vi "Doktorarbeit_Cornelius.vi"(0 "Heizer":refnum<visa-resource-name>="COM1", 1 "Setpoint\n START":bool, 2 "Write to File":bool, 3 "SP 1 shall be (°C)":dbl=20.0 min=0.0 max=999.0, 4 "Intervall (s)":u32 max=600, 5 "Write/\nRead":bool=TRUE, 6 "Delay (ms)":u32=500 min=100 max=600000, 7 "Auto Tune":bool, 9 "Standby":bool, 11 "Reset\nSTOPP":bool, 12 "Read Temperature":bool=TRUE, 13 "Get Values":bool, 15 "File Path":path) -> (8 "Temperature (°C)":dbl format="%#.3f", 14 "SP 1 is (°C)":dbl)   [LabVIEW 2010]
doc: "1. Verwendung\n\nDas Programm dient der Steuerung und Abfrage des Thermocontrollers I3252 und dem Auslesen von zwei VC 840 Messgeräten und einem Druckmessgerät Pfeiffer Single Gauge. \nDie Messgeräte werden Standardmäßig ausgelesen und erst nach Betätigung des Schalters \"Write to File\" in einer Textdatei abgespeichert. Das Eingabefeld \"Intervall\" legt den Abstand der Messpunkte fest.\nDer Setpoint für den Thermocontroller wird erst nach Betätigung des Tasters \"Setpoint START\" übernommen und angesteuert. Er wird ind den EEPROM des Gerätes geschrieben. Die Regelung kann mit Hilfe des Schalters \"Standby\" unterbrochen werden. Durch den Taster \"Reset STOPP\" kann der Setpoint aus dem EEPROM gelöscht werden.\nDie Eingabeflächen \"Constant\" und \"Thickness\" dienen der Berechnung des spezifischen Widerstands.\nDie Eingabeflächen \"User\" und \"Sample\" werden in den Header der Textdatei übernommen.\nDer Indikator \"File Path\" zeigt den aktuellen Speicherort der Textdatei an. Dieser wird nach ausschalten des Schalters \"Write to File\" gelöscht. Bei erneuten Schreiben muss ein neuer Speicherort gewählt werden. Bei Wahl desselben Speicherorts werden sämtliche bereits gespeicherte Daten gelöscht.\n\n\n2. Erläuterungen zum Blockdiagramm\n2.1 äußere Sequenz\nDie äußerte Sequenz besteht aus fünf Frames. Der erste dient der Initialisierung der Ports. Der zweite dient als Verzögerung um dem Programm genug Zeit zu geben die Ports zu öffnen. Jedoch senden die beiden VC 840 bereits Informationen an den Computer die in einem Puffer zwischengespeichert werden. Im dritten Frame wird dieser Puffer geleert. Somit kommt es zu keinem Framing Error. Desweiteren wird in diesem Frame die Startzeit der Messungen genommen. Im vierten Frame wird die eigentliche Messung und Verarbeitung der Daten durchgeführt. Die while-Schleife wird nur durch Auftreten eines Fehlers oder durch Betätigung des Stopbuttons auf dem Front Panel in der oberen linken Ecke unterbrochen. Im fünften und letzten Frame werden die Ports wieder geschlossen und beim Auftreten eines Fehlers wird das Programm automatisch gestoppt. Falls kein Fehler auftritt wird die Sequenz von vorne abgearbeitet.\n\n2.2 while-Schleife und innere Sequenz\n2.2.1 \"Event Structure\"\n2.2.1.1 Allgemein\nDer erste Frame beinhaltet ein \"Event Structure\". Dieser reagiert auf insgesamt elf verschiedene Ereignisse. Falls keines dieser Ereignisse auftreten sollte, warte die Struktur eine Millisekunde bevor die \"Event Structure\" verlassen wird. Die übrigen Ereignisse treten ein, wenn der entsprechende Kontroller eine Werteänderung erfährt.\n\n2.2.1.2 Event: Setpoint\nDieser Case besteht von außen nach innen aus einer Stacked Sequence, einer for-Loop und einer Flat Sequence die wiederum zwei \"Case Structures\" enthält. Als erstes wird bei dem Schalter \"Setpoint START\" der Blinkmodus aktiviert und bei dem Schalter \"Read Temperature\" deaktiviert. Danach folgt das eigentliche setzen des Temperatursollwerts. In der ersten Iteration wird dem Controller I3252 ein Schreibbefehl gesendet. Theoretisch kann der Setpoint in den RAM oder in den EEPROM geschrieben werden. Diese Auswahl erfolgt mit Hilfe des Schalters \"RAM\". Da das Schreiben in den RAM -Speicher aber aus diversen Gründen nicht erwünscht ist, wurde es nicht implementiert. Eine nachträgliche Implementierung ist aber leicht möglich, in dem die untere String-Konstante \"*P012\" durch \"*W012\" ersetzt wird. An diesem Befehl wird eine fünfstellige Hexadezimalzahl angehängt, die den Sollwert wiedergibt. Der Sollwert wird vorher mit zehn multipliziert, da das Komma standardmäßig nach der ersten Ziffer festgesetzt wurde (Bsp.: 800 wird gesendet um 80 einzustellen). Dieser Befehlsstrang wird an das Gerät mittels des SubVIs \"Comm_Interface\", auf welches später noch näher eingegangen wird, weitergegeben. Der durch das Gerät zurückgegebene String wird nicht verarbeitet.\nDie zweite Iteration dient dem Auslesen des eingestellten Sollwertes. Wahlweise kann der RAM- oder der EEPROM-Speicher ausgelesen werden. Die eigentliche Verarbeitung des Ausgabestrings erfolgt durch das SubVI \"Edit Setpoint\".\nDie Implementierung zur Einstellung des zweiten Setpoints erfolgt durch kopieren der ersten beiden Fälle und ersetzen der \"1\" im Befehf durch eine \"2\" (Bsp.: \"*P012\" zu \"*P022\"). Es darf aber nicht vergessen werden, dass dann ebenfalls die Anzahl der Iterationen angepasst werden muss.\nAls letztes wird der Blinkmodus des Schalters \"Setpoint START\" wieder deaktiviert.\n\n2.2.1.3 Event: Standby\nDieses Ereignis aktiviert bzw. deaktiviert als erstes den Blinckmodus des entsprechenden Schalters und sendet danach den Befehl zum aktivieren (\"*D03\") oder zum deaktivieren (\"*E03\") des Standbymodus an den Thermocontroller.\n\n2.2.1.4 Event: Set Command \nDer in das Feld \"Command shall be\" eingegebene Befehl wird an den Thermocontroller übermittlet. Die korrekte Form des Befehls ist im \"Communication Manuel\" nachzuschlagen. Das \"*\"-Zeichen wurde allerdings schon implementiert und muss somit nicht mit eingegeben werden.\n\n2.2.1.5 Event: Reset\nIn der ersten Iteration wird der Reset-Befehl an den Thermocontroller gesendet. In Folge wird der gesamte EEPROM-Speicher gelöscht. Deshalb wird in der zweiten Iteration der Setpoint aktualisiert. Dieser Befehl hat keinen Einfluss auf den RAM-Speicher. Die anschließende Wartezeit ist auf vier Sekunden festgesetzt und wurde empirisch ermittelt. Diese Zeit benötigt das Gerät um den Reset durchzuführen und für die Kommunikation wieder zur Verfügung zu stehen.\n\n2.2.1.6 Event: Auto Tune\nEs ist festgeschrieben, dass der Setpoint für die \"Auto Tune\"-Funktion wenigstens 20°C über der aktuellen Temperatur liegt. Deshalb wird zunächst der aktuelle Temperaturwert ausgelesen. Im zweiten Schritt werden zu diesem Wert zwanzig addiert und der Setpoint wird in den RAM-Speicher geschrieben. Das Schreiben in diesen Speicher ist nötig, da die \"Auto Tune\"-Funktion\" erst nach einem Reset startet. Im dritten Schritt wird der eigentliche Befehl für den \"Auto Tune\" gesendet (siehe dazu \"Communication Manuel\" S.27). Als vierte und letzte Iteration der for-Schleife folgt der bereits erwähnte Reset-Befehl. Der Temperatursollwert, der im RAM-Speicher eingetragen ist, muss zum Schluss wieder auf 0°C gesetzt werden. Die Zeit für die Ausführung des \"Auto Tune\"-Befehls wurde empirisch ermittelt und 45 s festgesetzt.\n\n2.2.1.7 Event: Write LOW/HI\nDieses Ereignis setzt die am Analogausgang anliegende Spannung fest. Normalerweise beträgt dieser Spannungswert 0-10 V. Das angeschlossene Netzteil verträgt aber maximal nur 2,3 V. Aus diesem Grund wird der \"%HIGH\" auf 23 gesetzt. Somit beträgt die maximal anliegende Spannung nur noch 23% von der maximal möglichen, d.h 2,3V. Ein niedrigerer Wert ist jederzeit möglich, genauso wie ein höherer für den Parameter \"%LOW\". Diese werden zunächst nacheinander in den RAM-Speicher geschrieben und anschließend wieder ausgelesen.\n\n2.2.1.8 Event: Set PID\nDie Werte für den PID-Regler können sowohl mit Hilfe der \"Auto Tune\"-Funktion, als auch manuell eingestellt werden. Es wird wiederum zwischen dem Schreiben in den RAM- und dem EEPROM-Speicher unterschieden. Zunächst werden die Werte für \"P\", \"I\" und \"D\", in dieser Reihenfolge, gesetzt und danach die aktuellen Werte ausgelesen.\n\n2.2.1.9 Event: Get Values\nDieses Ereignis hat zur Folge, dass die Werte für \"P\", \"I\", \"D\", \"%LOW\", \"%HIGH\" und des Setpoints wahlweise aus dem RAM- oder EEPROM-Speicher gelesen werden. Die aktuellen Werte werden nicht nur in die entsprechenden Anzeigefelder übernommen, sondern auch in die entsprechenden Eingabefelder, mit Ausnahme des Temperatursollwerts. \n\n2.2.1.10 Event: RAM\nPrinzipiell kann zwischen dem Schreiben in den RAM- oder EEPROM-Speicher des Thermocontrollers gewählt werden. Die entsprechende Schalterposition auf dem Frontpanel zeigt den aktuell verwendeten Speicher an. Die Anzeigewerte werden bei jedem Umschalten aktualisiert und sind im entsprechenden Speicher eingetragen. Die Implementierung ist identisch mit der des Ereignisses \"Get Values\". Es gilt zu beachten, dass die Werte für \"%LOW\" und \"%HIGH\" nur in den RAM-Speicher geschrieben werden können und somit auch nur aus diesem ausgelesen werden können.\n\n2.2.1.11 Event: Set Gauge to Zero\nMit Hilfe der SubVIs \"Get Pressure\" und \"Offset Display\" werden die Werte für den alten und den neuen Offset und der durch den zweiten Drucksensor ermittelt Druck ermittelt. \n\n2.2.1.12 Event: Write to File\nSollte der Schalter \"Write to File\" aktiviert werden, d.h. Schalterposition oben, so wird zunächst durch das SubVI \"Header\" ein Header für die unter \"File Path\" definierte Datei angelegt. Alle Werte, die bereits in der entsprechenden Datei stehen, werden dabei gelöscht.\n\n2.2.2 \"Timed Structures\"\nIm dritten Frame der inneren Sequenz werden die Werte für Zeitpunkt, Temperatur, Spannung, Strom und Druck ermittelt. Damit die Werte zum gleichen Zeitpunkt aufgenommen werden, werden \"Timed Sequences\" eingesetzt. Mit dem entsprechenden Schalter auf dem Front Panel unter dem Tab \"Settings\" kann gewählt werden, ob das entsprechende Gerät ausgelesen werden soll oder nicht. Die einzelnen Sequenzen werden parallel abgearbeitet, womit die Prozesszeit von diesem Frame durch der zeitintensivsten Sequenz abhängt. Dies ist in aller Regel das Auslesen der Temperatur, da ein \"Delay\" von 500 ms oder größer benötigt wird, um den Controller ordentlich ansprechen zu können.\nDie Systemzeit wird durch das SubVI \"System Time in Seconds\" in Sekunden umgerechnet und der in dem Parameter \"Starttime\" gespeicherte Wert wird abgezogen. Somit werden die Sekunden seit dem Start des Programms gezählt.\n\n2.2.3 restlichen Frames\nIm zweiten Frame wird das Intervall zwischen den einzelnen Messwerten festgelegt. Dabei wird der Wert des Parameters \"Delay\" abgezogen. Dieser Wert beträgt im Normalfall 500 ms und ist somit nicht vernachlääsigbar.\nDer Vierte Frame beinhaltet die Umrechnung des Temperatur-Strings in einen Temperaturwert durch das SubVI \"Edit Tmperature\", die Berechnung des spezifischen Widerstands durch das SubVI \"Resistivity Calculation\" und die Überprüfung des Druckwerts. Auch werden die neu gewonnen Werte in das entsprechende Shift-Register übernommen. Falls der Druckwert einen in dem Parameter \"Pressure Limit (mbar)\" festgelegten Grenzwert überschreiten sollte, wird der Thermocontroller automatisch in den Standby-Modus versetzt. Des Weiteren wird der Schalter \"Standby\" solange gesperrt, wie der Druck oberhalb des Grenzwertes liegt. Wenn der Druck wieder unter den Grenzwert gesunken ist, wird der Standby-Befehl nicht automatisch aufgehoben, sondern muss vom Benutzer durch Betätigung des entsprechenden Schalters gegeben werden.\nIm fünften Frame werden die Diagramme erstellt. Dabei wird jedes Mal von neuem das gesamte Shift-Register als Graph dargestellt. Weiterhin werden die Messwerte in ein 1D-Array geschrieben.\nDer sechste und letzte Frame beinhaltet den eigentlich Schreibvorgang der Messwerte in eine Textdatei und die Überprüfung ob ein Fehler vorliegt.\n\n2.3 SubVIs\n2.3.1 Allgemein\nDie SubVIs für die Messgeräte VC840 und das Druckmessgerät wurden aus anderen Quellen übernommen. \n\n2.3.2 \"Header\"\nIn den Header wird zunächst das aktuelle Datum und die aktuelle Zeit übernommen. Die ausgewählte Datei wird dabei überschrieben. Danach wird der Name des Benutzers und der Probe übernommen. Zum Schluss werden die Einheiten in einer Reihe, durch einen Tabulator getrennt, in den Header geschrieben.\n\n2.3.3 \"I3252 Comm Interface\"\nDieses VI stellt die Kommunikation mit dem Thermocontroller her und gibt den Ausgabe-String zurück.\n\n2.3.4 \"I3252 Edit Setpoint\"\nIm Ausgabe-String vom Thermocontroller ist an der vierten Stelle die Stelle des Dezimalpunktes verschlüsselt. Dieses Hexadezimalzahl wird herausgefiltert und an ein \"ENUM Controller\" übergeben. Dieser weist der Hexadezimalzahl eine Nummer zu, mit welcher ein Wert aus einem Array entnommen wird. Dieser Wert dient als Quotient. Der tatsächliche Wert kann somit errechnet werden.\n\n2.3.5 \"I3252 Edit Temperature\"\nDer Temperatur-String, der vom Thermocontroller zurückgegeben wird, wird in eine Dezimalzahl umgewandelt. Manchmal kommt es aus zu Dropouts, die durch dieses Programm herausgefiltert werden. Der letzte Wert wird dabei in einer \"Feedback Node\" gehalten unter der Annahme, dass sich der Temperaturwert nicht sprunghaft ändert.\n\n2.3.6 \"Resistivity Calculation\"\nDer spezifische Widerstand wird nach folgender Formel ausgerechnet. Dabei entspricht t der Dicke der Probe und C ist eine Konstante.\nrho=C*pi*t*U/(ln( 2)*I)\n\n2.3.7 \"System Time in Seconds\"\nZunächst wird die aktuelle Systemzeit ausgelesen. Danach wird diese in Stunden, Minuten und Sekunden aufgeteilt, alles in Sekunden umgerechnet und letztendlich addiert."
uses:
  <vilib>/Platform/TimedLoop/XDataNode/XDataNode.xnode
  <vilib>/Platform/TimedLoop/XDataNode/timing_clust.ctl
  <vilib>/Platform/TimedLoop/XDataNode/nitl_modes.ctl
  <vilib>/Platform/TimedLoop/XDataNode/wakeup.ctl
  <vilib>/Instr/_visa.llb/VISA Configure Serial Port (Instr).vi
  <vilib>/Platform/TimedLoop/scheduler/LVUserAPI/_suppVIs/Create_1kHz_TSource.vi
  <vilib>/Utility/file.llb/Write To Spreadsheet File (DBL).vi
  <vilib>/Platform/TimedLoop/XDataNode/XDNodeRunTimeDep.lvlib
panel:
  out "appended array":dbl[](array[numeric])
  in  "Tab Control":T1(tab)
  out "Pressure":cluster{dbl[], dbl[]}(graph)
  out "Pressure (mbar)":dbl format="%.2e"
  in  "Thickness (nm)":dbl min=0.0
  in  "Constant":dbl=4.532 min=0.0 max=5.0
  in  "Sample":string
  in  "User":string
  out "Temperature":cluster{dbl[], dbl[]}(graph)
  out "Resistivity":cluster{dbl[], dbl[]}(graph)
  out "Resistivity (Ohm*cm)":dbl format="%.3e"
  out "time (s)":dbl
  in  "Pressure Limit (mbar)":dbl=0.0001 min=0.0 max=1100.0
  out "Pressure 1 (mbar)":dbl
  out "Current Offset (mbar)":dbl
  out "Old Offset (mbar)":dbl
  out "Pressure 2 (mbar)":dbl
  out "Status":T2(ring)
  in  "Sensor Nr.:":enum16{"sensor 1", "aensor 2", "test"}(ring)
  in  "Port":T3(ring)=enum."COM 5"
  in  "Set Gauge to Zero":bool
  out "Error Out":bool
  in  "VC 840 2":refnum<visa-resource-name>="COM4"
  out "Reading 2":dbl format="%_4f"
  out "Mode 2":enum16{"?", "Diode", "Beep", "DC", "AC"}(ring)
  out "Unit 2":string
  in  "VC 840 1":refnum<visa-resource-name>="COM3"
  out "Reading 1":dbl format="%_4f"
  out "Mode 1":enum16{"?", "Diode", "Beep", "DC", "AC"}(ring)
  out "Unit 1":string
  out "Status 1":T4
  out "Status 2":T4
  in  "Set Command":bool
  in  "Set PID":bool
  in  "Write LOW/HI":bool
  out "% HIGH is":u32
  out "% LOW is":u32
  in  "% High shall be":u32=23 max=24
  in  "% LOW shall be":u32 max=25
  in  "Flow Control":u16(ring) items=["None"=0, "XON/XOFF"=1, "RTS/CTS"=2, "DTR/DSR"=4]
  in  "Stop Bits":u16(ring)=10 items=["1.0"=10, "1.5"=15, "2.0"=20]
  in  "Parity":u16(ring)=1 items=["None", "Odd", "Even", "Mark", "Space"]
  in  "Data Bits":u16=7 min=5 max=8 step=1
  in  "Baud Rate":u32=9600
  out "Command is":string
  in  "Command shall be":string
  in  "RAM":bool=TRUE caption="EEPROM"
  out "D (Rate) is":u32
  out "I ( Reset1) is":u32
  out "P (PB1) is":u32
  in  "D (Rate) shall be":u32 max=3999
  in  "I ( Reset1) shall be":u32 max=3999
  in  "P (PB1) shall be":u32 max=9999
  in  "Read VC 840 1":bool=TRUE
  in  "Read VC 840 2":bool=TRUE
  in  "Read Pressure":bool=TRUE
  out "Starttime":dbl
  out "Current":cluster{dbl[], dbl[]}(graph)
  out "Voltage":cluster{dbl[], dbl[]}(graph)
  out "Voltage (V)":dbl format="%.4e"
  out "Current (A)":dbl format="%.4e"
  # "I3252 Control"
  # "VC 840 Control"
  # "Pfeiffer Control"
  # "Authors:  Daniel Schuster (sir-dan@web.de)\n                 Steffen Cornelius (s.cornelius@hzdr.de)\n\n                 premade SubVIs for readout of Pfeiffer gauge and VC840 Multimeters were used\n                 SubVI \"I3252_Comm_Interface\" is based on a modified Labview example\n\nRelease:  v1.0    \n\nVersion History:\n\nv1.1  28.06.2011\n             - Format des Files geändert von %.3f auf %g\n             - maximale Eingabewerte für PID begrenzt\nv1.2  12.07.2011\n             - Anzeige p,rho, U, V auf Scientific geändert\n             - y-Achse p,rho auf Log geändert\n             - numerische Zeitanzeige hinzugefügt\n             - 4PP Constant: pi/ln(2)=4,532 set as the default value\nv1.3  25.07.2011\n             - Zeitvariable auf EXT geändert, um Sprünge in Diagrammen loszuwerden"
  # "Version 1.3    - last change 25.07.2011"
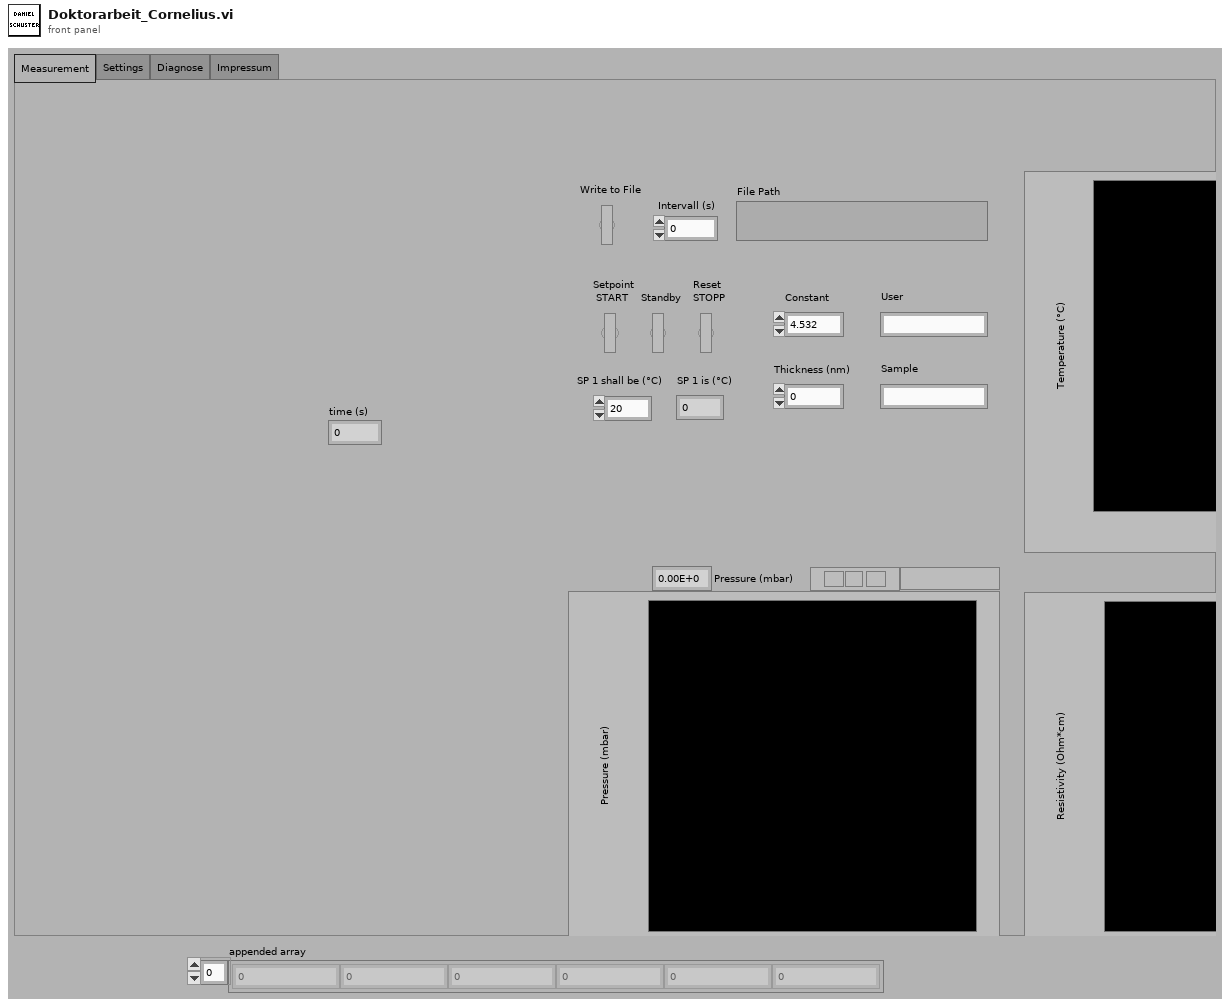
[diagram p1: front panel]
types:
  T1 = enum32{"Measurement", "Settings", "Diagnose", "Impressum"}
  T2 = enum16{"data OK", "underrange", "overrange", "sensor error", "sensor off", "no sensor", "ID error"}
  T3 = enum16{"COM 1", "COM 2", "COM 3", "COM 4", "COM 5", "COM 6", "COM 7", "COM 8", "COM 9", "COM 10", "COM 11", "COM 12"}
  T4 = cluster{"Low Bat":bool, "Auto":bool, "Delta":bool, "Hold":bool, "RS232":bool}
  T5 = typedef "XDNodeRunTimeDep.lvlib/timing_clust.ctl" = cluster{"Expected End [f-1]":u64, "Actual End [f-1]":u64, "Finished Late? [f-1]":bool, "Expected End [i-1]":u64, "Actual End [i-1]":u64, "Finished Late? [i-1]":bool, "Expected Start [i]":u64, "Actual Start [i]":u64, "Expected Start [f]":u64, "Actual Start [f]":u64, "Source Name":string, "Structure Name":string, "Period":i64, "Deadline":i64, "Offset":i64, "Start":i64, "Priority":i32, "Timeout":i32, "Mode":T6, "Wakeup Reason":T7, "Error":errorcluster, "Source Type":string, "Secondary Source Type":string, "Global End Time":u64, "Global Start Time":u64, "Frame Duration":u64, "Iteration Duration":u64, "Assigned CPU":i32, "I/O Scan Engine Mode":u32}
  T6 = typedef "XDNodeRunTimeDep.lvlib/nitl_modes.ctl" = enum32{"No Change", "Process missed periods, maintain original phase", "Discard missed periods, maintain original phase", "Process missed periods, ignore original phase", "Discard missed periods, ignore original phase"}
  T7 = typedef "XDNodeRunTimeDep.lvlib/wakeup.ctl" = enum32{"Normal", "Aborted", "Asynchronous wakeup", "Timing source error", "Timed loop error", "Timeout"}
  T8 = enum8{"Enabled", "Disabled", "Disabled and Grayed Out"}
  T9 = cluster{"VISA resource name out":refnum<visa-resource-name>, "error out":errorcluster, "Delay (ms)":u32, "Write/\nRead":bool}
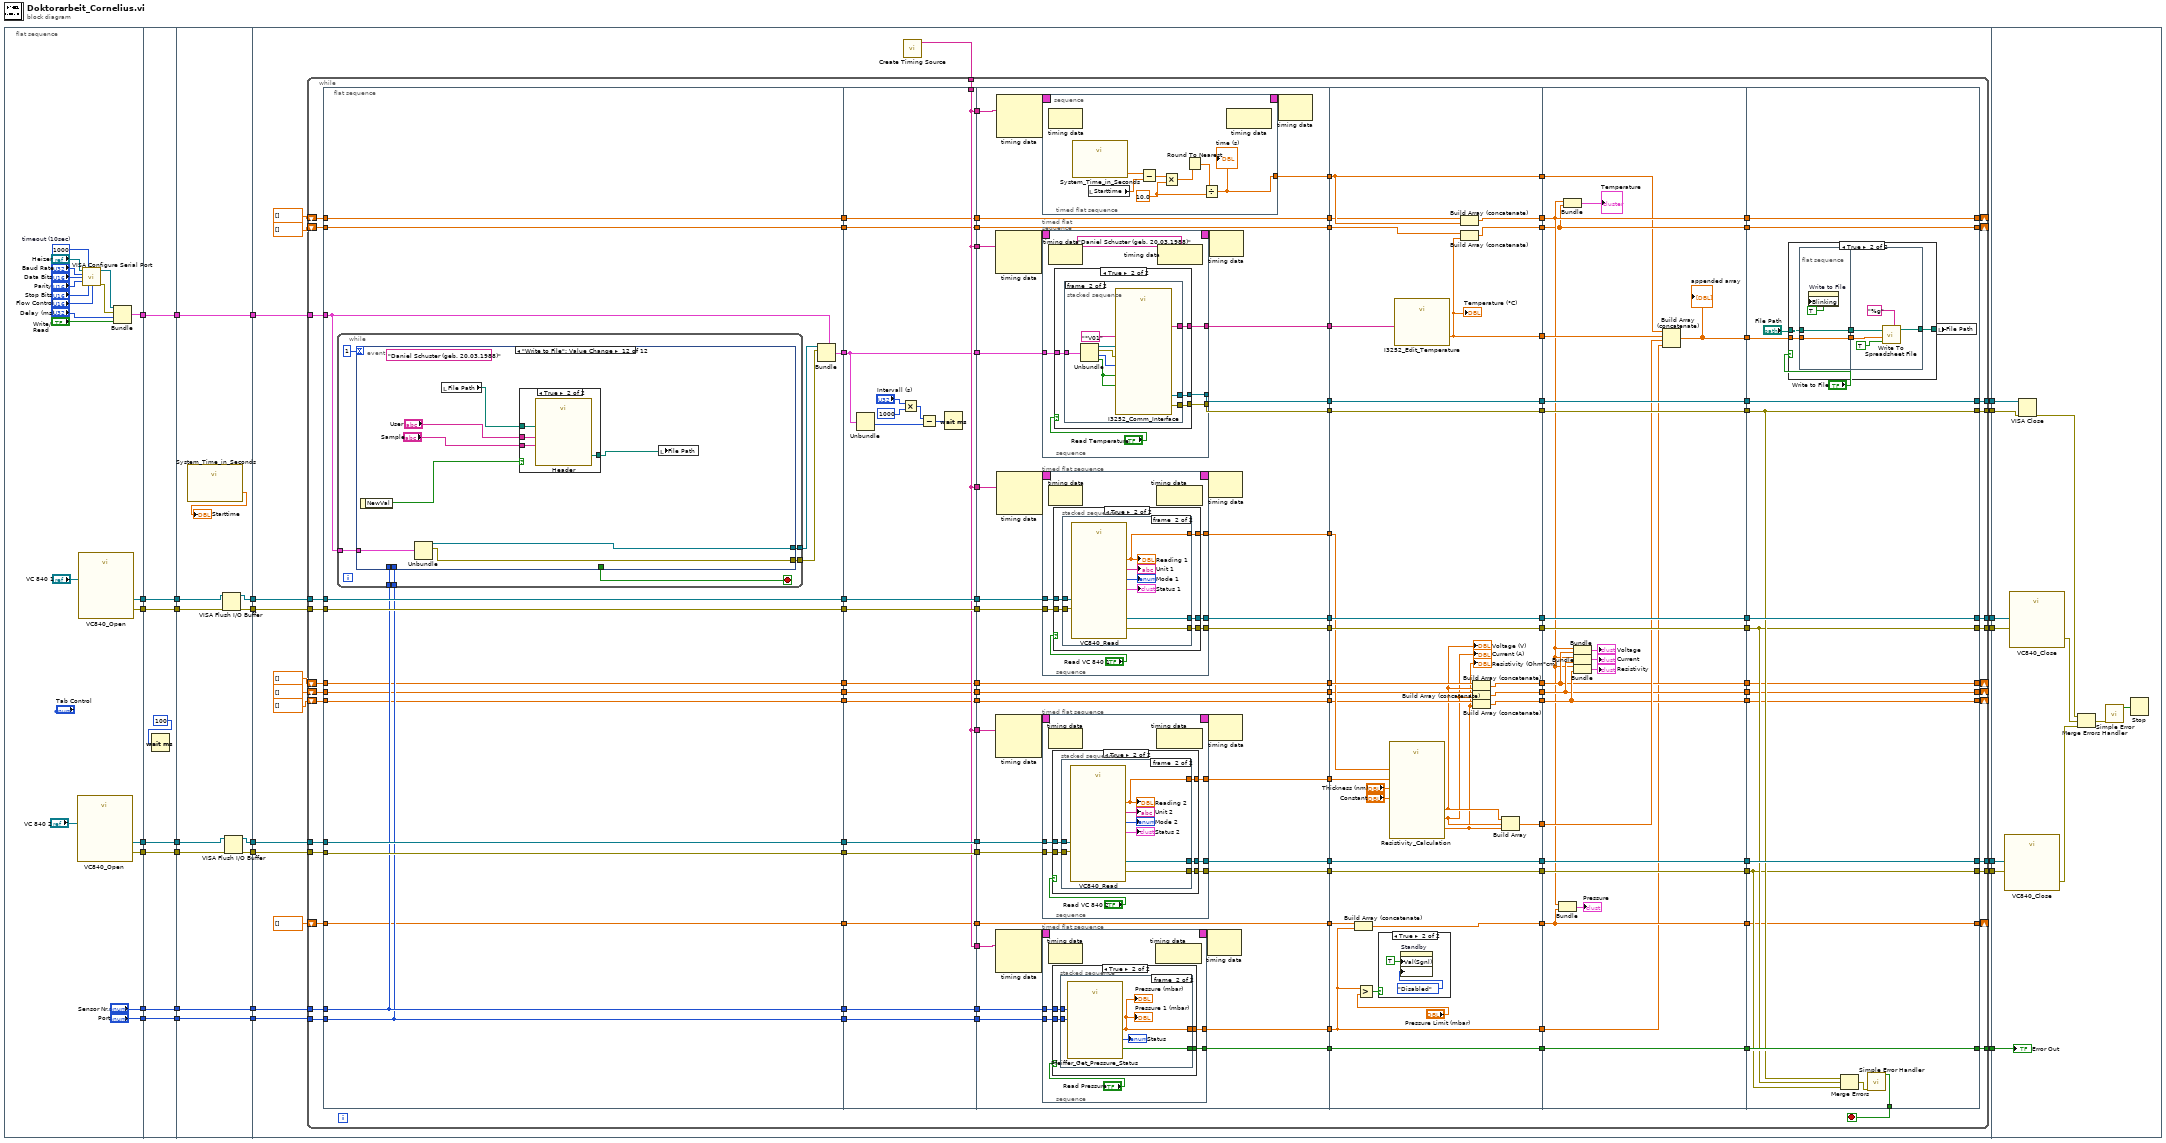
[diagram p0: block diagram]
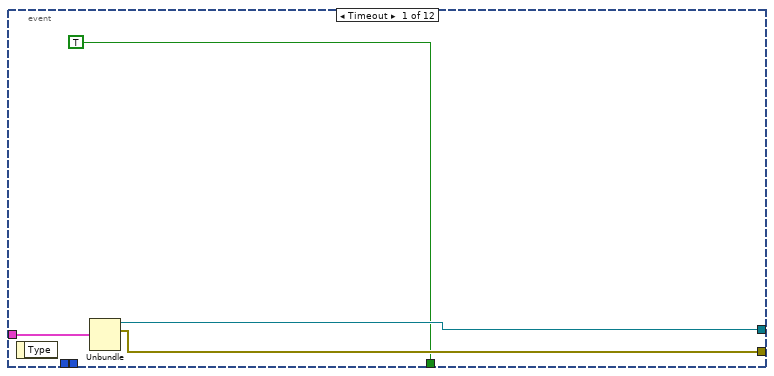
[diagram p2: hidden frame]
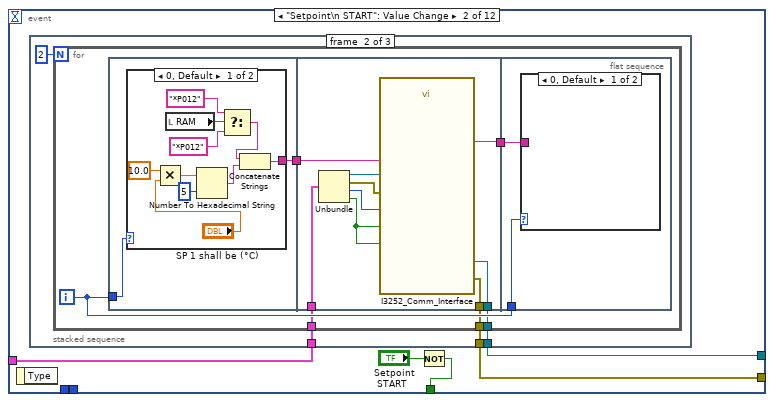
[diagram p3: hidden frame]
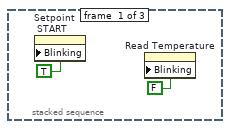
[diagram p4: hidden frame]
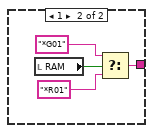
[diagram p5: hidden frame]
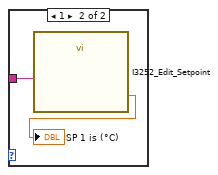
[diagram p6: hidden frame]
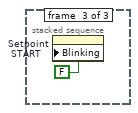
[diagram p7: hidden frame]
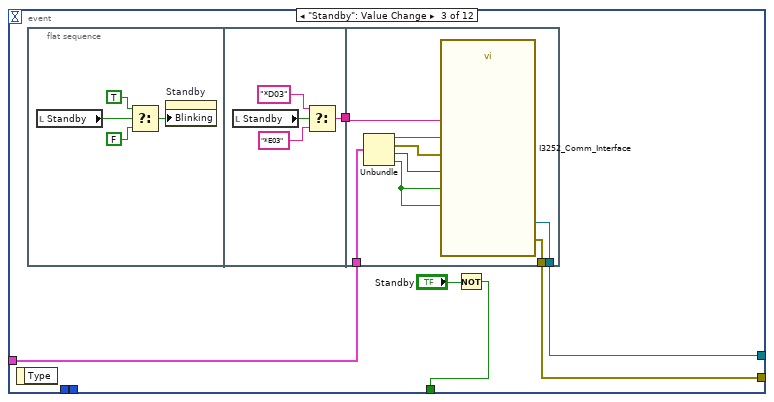
[diagram p8: hidden frame]
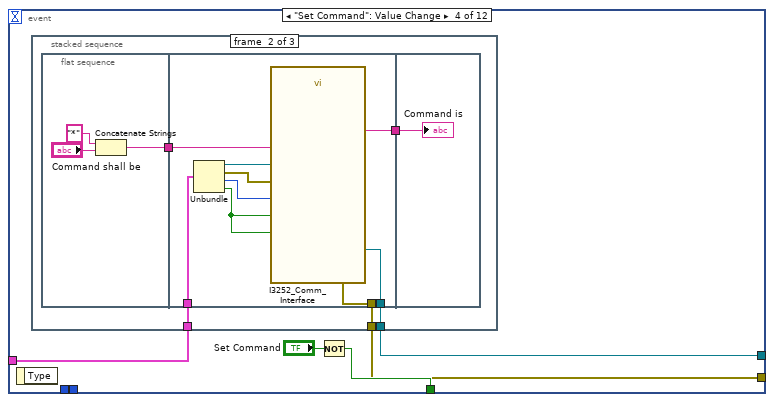
[diagram p9: hidden frame]
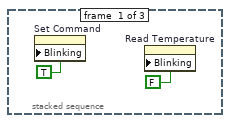
[diagram p10: hidden frame]
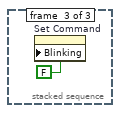
[diagram p11: hidden frame]
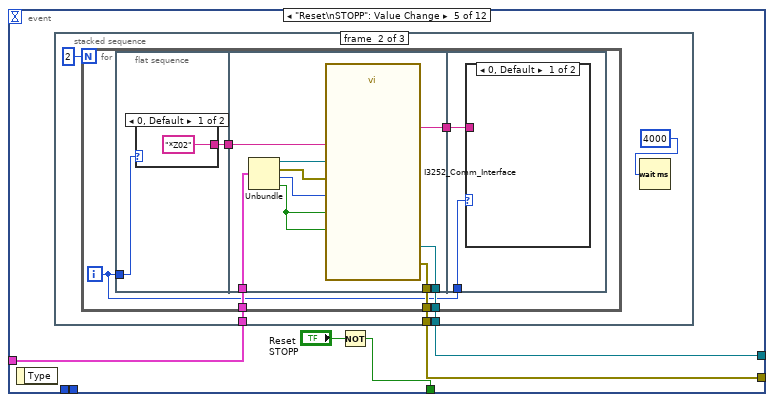
[diagram p12: hidden frame]
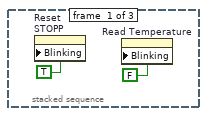
[diagram p13: hidden frame]
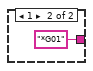
[diagram p14: hidden frame]
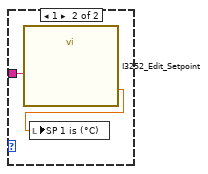
[diagram p15: hidden frame]
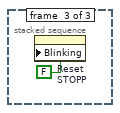
[diagram p16: hidden frame]
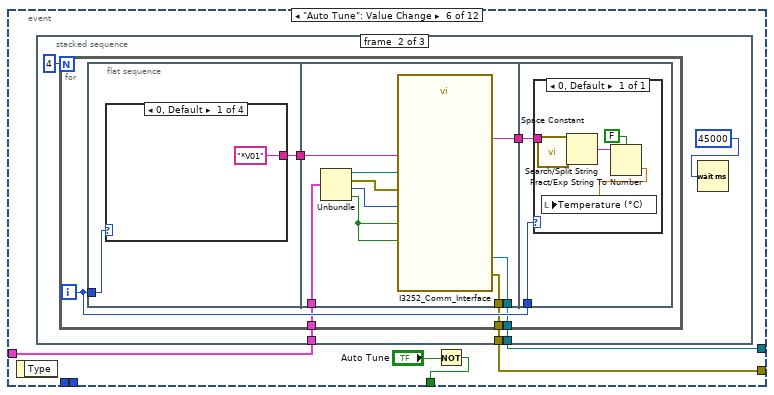
[diagram p17: hidden frame]
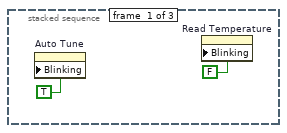
[diagram p18: hidden frame]
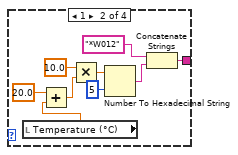
[diagram p19: hidden frame]
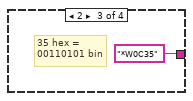
[diagram p20: hidden frame]
diagram:
  n1 = flat-sequence {
    tunnel: [w47] -> w21
    tunnel: [w48] -> w20
    tunnel: [w31] -> w19
    tunnel: [w46] -> w18
    tunnel: [w45] -> w17
    tunnel: ["Port"] -> w16
    tunnel: ["Sensor Nr.:"] -> w15
    tunnel: w21 -> [w56]
    tunnel: [w56] -> w14
    tunnel: w20 -> [w55]
    tunnel: [w55] -> w12
    tunnel: w19 -> [w54]
    tunnel: [w54] -> w10
    tunnel: w18 -> [w53]
    tunnel: [w53] -> w8
    tunnel: w17 -> [w52]
    tunnel: [w52] -> w6
    tunnel: w16 -> [w51]
    tunnel: [w51] -> w4
    tunnel: w15 -> [w50]
    tunnel: [w50] -> w2
    tunnel: w14 -> [w60]
    tunnel: [w59] -> w13
    tunnel: w12 -> [w61]
    tunnel: [w58] -> w11
    tunnel: w10 -> [w68]
    tunnel: [w68] -> w9
    tunnel: w8 -> [w63]
    tunnel: [w64] -> w7
    tunnel: w6 -> [w62]
    tunnel: [w65] -> w5
    tunnel: w4 -> [w67]
    tunnel: [w67] -> w3
    tunnel: w2 -> [w66]
    tunnel: [w66] -> w1
    tunnel: w13 -> [w89]
    tunnel: w11 -> [w88]
    tunnel: w9 -> [w87]
    tunnel: w7 -> [w85]
    tunnel: w5 -> [w84]
    tunnel: w3 -> [w77]
    tunnel: w1 -> [w76]
    tunnel: [w83] -> w28
    tunnel: [w82] -> w27
    tunnel: [w81] -> w26
    tunnel: [w80] -> w25
    tunnel: [w79] -> w24
    tunnel: [w78] -> w23
    tunnel: [w75] -> w22
    tunnel: w28 -> [w1023]
    tunnel: w27 -> [w1022]
    tunnel: w26 -> [w1025]
    tunnel: w25 -> [w1024]
    tunnel: w24 -> [w1027]
    tunnel: w23 -> [w1026]
    tunnel: w22 -> [w1021]
    frame #0 {
      w32 = u32 1000  # timeout (10sec)
      n2 = call "VC840_Open.vi"("VISA resource name"="VC 840 2") -> ("error out"=w45:errorcluster, "VISA resource name out"=w46:refnum<visa-resource-name>)  [unwired: 1 in, 8 out]
      n3 = call "VC840_Open.vi"("VISA resource name"="VC 840 1") -> ("error out"=w48:errorcluster, "VISA resource name out"=w47:refnum<visa-resource-name>)  [unwired: 1 in, 8 out]
      n4 = call-poly "VISA Configure Serial Port"("VISA resource name"="Heizer", "timeout (10sec)"=w32, "baud rate (9600)"="Baud Rate", "data bits (8)"="Data Bits", "parity (0:none)"="Parity", "stop bits (10: 1 bit)"="Stop Bits", "flow control (0:none)"="Flow Control") -> ("VISA resource name out"=w41:refnum<visa-resource-name>, "error out"=w42:errorcluster)  [unwired: 2 in, 5 out]
      n5 = Bundle("VISA resource name out"=w41, "error out"=w42, "Delay (ms)"="Delay (ms)", "Write/\nRead"="Write/\nRead") -> (w31:T9)  [unwired: 1 in]
    }
    frame #1 {
      n6 = Wait (ms)(milliseconds to wait=u32 100) -> ()  [unwired: 1 out]
    }
    frame #2 {
      n7 = call "System_Time_in_Seconds.vi"() -> ("Current Time (s)"=→"Starttime":dbl)
      n8 = VISA Flush I/O Buffer(VISA resource name=w60, error in (no error)=w61) -> (VISA resource name out=w59:refnum<visa-resource-name>, error out=w58:errorcluster)  [unwired: 1 in]
      n9 = VISA Flush I/O Buffer(VISA resource name=w63, error in (no error)=w62) -> (VISA resource name out=w64:refnum<visa-resource-name>, error out=w65:errorcluster)  [unwired: 1 in]
    }
    frame #3 {
      n10 = call-poly <vilib>:"Create Timing Source.vi"() -> ("name (out)"=w86:string)  [unwired: 10 in, 1 out]
      n11 = while {
        tunnel: w89 -> [w197]
        tunnel: w88 -> [w196]
        tunnel: w87 -> [w195]
        tunnel: w86 -> [w187]
        tunnel: w85 -> [w180]
        tunnel: w84 -> [w179]
        tunnel: [w175] -> w83
        tunnel: [w174] -> w82
        tunnel: [w172] -> w81
        tunnel: [w170] -> w80
        tunnel: [w168] -> w79
        tunnel: [w166] -> w78
        tunnel: w76 -> [w162]
        tunnel: w77 -> [w160]
        tunnel: [w158] -> w75
        shift-right: [w124] -> _
        shift-left: dbl[] [] -> [w129]
        shift-right: [w100] -> _
        shift-left: dbl[] [] -> [w143]
        shift-right: [w126] -> _
        shift-left: dbl[] [] -> [w133]
        shift-right: [w97] -> _
        shift-left: dbl[] [] -> [w142]
        shift-right: [w136] -> _
        shift-left: dbl[] [] -> [w139]
        shift-right: [w94] -> _
        shift-left: dbl[] [] -> [w141]
        stop <- w90 stop-if-true
        n12 = flat-sequence {
          tunnel: w195 -> [w211]
          tunnel: w196 -> [w212]
          tunnel: w197 -> [w213]
          tunnel: [w213] -> w194
          tunnel: [w212] -> w192
          tunnel: [w208] -> w190
          tunnel: w180 -> [w207]
          tunnel: [w207] -> w184
          tunnel: w179 -> [w206]
          tunnel: [w206] -> w182
          tunnel: w162 -> [w205]
          tunnel: [w205] -> w161
          tunnel: w160 -> [w204]
          tunnel: [w204] -> w159
          tunnel: w143 -> [w200]
          tunnel: w142 -> [w199]
          tunnel: w141 -> [w198]
          tunnel: [w203] -> w140
          tunnel: w139 -> [w203]
          tunnel: [w202] -> w134
          tunnel: w133 -> [w202]
          tunnel: [w201] -> w130
          tunnel: w129 -> [w201]
          tunnel: [w200] -> w108
          tunnel: [w199] -> w105
          tunnel: [w198] -> w103
          tunnel: w194 -> [w743]
          tunnel: [w743] -> w193
          tunnel: w192 -> [w742]
          tunnel: [w742] -> w191
          tunnel: w190 -> [w735]
          tunnel: [w735] -> w189
          tunnel: [w737] -> w188
          tunnel: w187 -> [w737]
          tunnel: [w737] -> w186
          tunnel: [w737] -> w185
          tunnel: w184 -> [w741]
          tunnel: [w741] -> w183
          tunnel: w182 -> [w740]
          tunnel: [w740] -> w181
          tunnel: [w737] -> w178
          tunnel: [w739] -> w164
          tunnel: [w738] -> w163
          tunnel: w161 -> [w739]
          tunnel: w159 -> [w738]
          tunnel: [w737] -> w156
          tunnel: w140 -> [w730]
          tunnel: [w730] -> w137
          tunnel: w134 -> [w729]
          tunnel: [w729] -> w132
          tunnel: w130 -> [w728]
          tunnel: [w728] -> w127
          tunnel: [w727] -> w109
          tunnel: w108 -> [w727]
          tunnel: [w726] -> w106
          tunnel: w105 -> [w726]
          tunnel: [w725] -> w104
          tunnel: w103 -> [w725]
          tunnel: [w754] -> w155
          tunnel: w193 -> [w781]
          tunnel: w191 -> [w780]
          tunnel: w189 -> [w775]
          tunnel: w188 -> [w774]
          tunnel: w186 -> [w773]
          tunnel: w185 -> [w772]
          tunnel: w183 -> [w759]
          tunnel: w181 -> [w758]
          tunnel: w178 -> [w760]
          tunnel: [w756] -> w154
          tunnel: [w757] -> w153
          tunnel: [w771] -> w152
          tunnel: [w770] -> w151
          tunnel: [w769] -> w150
          tunnel: [w768] -> w149
          tunnel: w164 -> [w767]
          tunnel: w163 -> [w766]
          tunnel: [w763] -> w148
          tunnel: w156 -> [w755]
          tunnel: [w753] -> w147
          tunnel: [w752] -> w146
          tunnel: [w751] -> w145
          tunnel: [w750] -> w144
          tunnel: [w749] -> w138
          tunnel: w137 -> [w749]
          tunnel: w132 -> [w748]
          tunnel: [w748] -> w131
          tunnel: [w747] -> w128
          tunnel: w127 -> [w747]
          tunnel: w109 -> [w746]
          tunnel: [w746] -> w107
          tunnel: w106 -> [w745]
          tunnel: w104 -> [w744]
          tunnel: [w745] -> w102
          tunnel: [w744] -> w101
          tunnel: w155 -> [w944]
          tunnel: [w941] -> w122
          tunnel: w154 -> [w960]
          tunnel: [w960] -> w121
          tunnel: w153 -> [w959]
          tunnel: [w959] -> w120
          tunnel: w152 -> [w958]
          tunnel: [w958] -> w119
          tunnel: w151 -> [w957]
          tunnel: [w957] -> w118
          tunnel: w150 -> [w956]
          tunnel: [w956] -> w117
          tunnel: w149 -> [w955]
          tunnel: [w955] -> w116
          tunnel: [w946] -> w115
          tunnel: w148 -> [w954]
          tunnel: [w954] -> w114
          tunnel: w147 -> [w938]
          tunnel: w146 -> [w948]
          tunnel: w145 -> [w946]
          tunnel: w144 -> [w949]
          tunnel: [w944] -> w113
          tunnel: w138 -> [w947]
          tunnel: [w945] -> w112
          tunnel: w131 -> [w943]
          tunnel: w128 -> [w942]
          tunnel: [w940] -> w111
          tunnel: [w928] -> w110
          tunnel: w107 -> [w939]
          tunnel: w102 -> [w936]
          tunnel: w101 -> [w935]
          tunnel: [w937] -> w98
          tunnel: [w934] -> w95
          tunnel: [w933] -> w92
          tunnel: [w929] -> w91
          tunnel: w122 -> [w978]
          tunnel: [w986] -> w177
          tunnel: [w985] -> w176
          tunnel: w121 -> [w985]
          tunnel: [w979] -> w173
          tunnel: w120 -> [w979]
          tunnel: [w984] -> w171
          tunnel: w119 -> [w984]
          tunnel: [w983] -> w169
          tunnel: w118 -> [w983]
          tunnel: [w982] -> w167
          tunnel: w117 -> [w982]
          tunnel: [w981] -> w165
          tunnel: w116 -> [w981]
          tunnel: w115 -> [w964]
          tunnel: [w980] -> w157
          tunnel: w114 -> [w980]
          tunnel: w113 -> [w965]
          tunnel: w112 -> [w976]
          tunnel: [w976] -> w135
          tunnel: w111 -> [w967]
          tunnel: [w967] -> w125
          tunnel: w110 -> [w966]
          tunnel: [w966] -> w123
          tunnel: [w969] -> w99
          tunnel: w98 -> [w969]
          tunnel: [w970] -> w96
          tunnel: w95 -> [w970]
          tunnel: [w971] -> w93
          tunnel: w92 -> [w971]
          tunnel: w91 -> [w977]
          tunnel: w177 -> [w988]
          tunnel: [w1005] -> w175
          tunnel: w176 -> [w1005]
          tunnel: [w998] -> w174
          tunnel: w173 -> [w998]
          tunnel: [w1004] -> w172
          tunnel: w171 -> [w1004]
          tunnel: [w1000] -> w170
          tunnel: w169 -> [w1000]
          tunnel: [w1003] -> w168
          tunnel: w167 -> [w1003]
          tunnel: [w1001] -> w166
          tunnel: w165 -> [w1001]
          tunnel: [w1002] -> w158
          tunnel: w157 -> [w1002]
          tunnel: [w994] -> w136
          tunnel: w135 -> [w994]
          tunnel: [w993] -> w126
          tunnel: w125 -> [w993]
          tunnel: [w992] -> w124
          tunnel: w123 -> [w992]
          tunnel: [w991] -> w100
          tunnel: w99 -> [w991]
          tunnel: [w990] -> w97
          tunnel: w96 -> [w990]
          tunnel: [w989] -> w94
          tunnel: w93 -> [w989]
          tunnel: [w987] -> w90
          frame #0 {
            n13 = while {
              tunnel: w211 -> [w219]
              tunnel: [w218] -> w210
              tunnel: [w217] -> w209
              tunnel: w205 -> [w216]
              tunnel: w204 -> [w215]
              stop <- w220 stop-if-true
              (unwired) "Daniel Schuster (geb. 20.03.1988)"
              n14 = event shown="[11] \"Write to File\": Value Change" {
                selector: _ -> [_ _ _ _ _ _ _ _ _ _ _ _]
                dyn-events: _ -> [_ _ _ _ _ _ _ _ _ _ _ _]
                timeout: 1 -> [_ _ _ _ _ _ _ _ _ _ _ _]
                tunnel: [TRUE ("Set Gauge to Zero") w228 w277 w298 w324 w359 w415 w466 w545 w616 "Set Gauge to Zero" _] -> w220
                tunnel: w219 -> [w224 w227 w274 w296 w320 w358 w411 w464 w543 w614 w693 w719]
                tunnel: [w223 w226 w273 w295 w322 w356 w413 w463 w542 w613 w692 w718] -> w218
                tunnel: [w222 w225 w272 w294 w321 w357 w412 w462 w541 w612 w691 w717] -> w217
                tunnel: w216 -> [_ _ _ _ _ _ _ _ _ _ w694 _]
                tunnel: w215 -> [_ _ _ _ _ _ _ _ _ _ w687 _]
                event Timeout {
                  n15 = event-data() -> ()  [unwired: 1 in, 1 out]
                  n16 = Unbundle(w224) -> ("VISA resource name out"=w223:refnum<visa-resource-name>, "error out"=w222:errorcluster)  [unwired: 2 out]
                }
                event "Setpoint\n START": Value Change {
                  n17 = event-data() -> ()  [unwired: 1 in, 1 out]
                  n18 = stacked-sequence {
                    tunnel: w227 -> [_ w234 _]
                    tunnel: [_ w233 _] -> w225
                    tunnel: [_ w232 _] -> w226
                    frame #0 {
                      n19 = property on="Setpoint\n START" class="Bool"("Blinking"=TRUE) -> ()  [unwired: 2 in, 2 out]
                      n20 = property on="Read Temperature" class="Bool (strict)"("Blinking"=FALSE) -> ()  [unwired: 2 in, 2 out]
                    }
                    frame #1 {
                      n21 = for {
                        N: 2 -> [_]
                        tunnel: w234 -> [w238]
                        tunnel: [w237] -> w233
                        tunnel: [w236] -> w232
                        i -> [w240]
                        n22 = flat-sequence {
                          tunnel: [w243] -> w239
                          tunnel: w240 -> [w242]
                          tunnel: [w261] -> w241
                          tunnel: w239 -> [w260]
                          tunnel: w238 -> [w262]
                          tunnel: [w259] -> w237
                          tunnel: [w258] -> w236
                          tunnel: w241 -> [w268]
                          tunnel: w240 -> [w267]
                          frame #0 {
                            n23 = case shown="0, Default" w242 {
                              tunnel: [w252 w254] -> w243
                              frame 0, Default {
                                n24 = Multiply(x=10.0, y="SP 1 shall be (°C)") -> (x*y=w249:dbl)
                                n25 = local read "RAM"() -> (w247:bool)
                                n26 = Number To Hexadecimal String(1:i16 5 ("width (-)"), 2:w249) -> (0:w251:string)
                                n27 = Select(t="*P012", s=w247, f="*P012") -> (s? t:f=w244:string)
                                n28 = Concatenate Strings(w244, w251) -> (w252:string)
                              }
                              frame 1 {
                                n29 = local read "RAM"() -> (w257:bool)
                                n30 = Select(t="*G01", s=w257, f="*R01") -> (s? t:f=w254:string)
                              }
                            }
                          }
                          frame #1 {
                            n31 = Unbundle(w262) -> ("VISA resource name out"=w263:refnum<visa-resource-name>, "error out"=w265:errorcluster, "Delay (ms)"=w264:u32, "Write/\nRead"=w266:bool)
                            n32 = call "I3252_Comm_Interface.vi"("VISA resource name in"=w263, "error in"=w265, "Delay (ms)"=w264, "Write"=w266, "String to Write"=w260, "Read"=w266) -> ("VISA resource name out"=w258:refnum<visa-resource-name>, "error out"=w259:errorcluster, "Read String"=w261:string)  [unwired: 2 in]
                          }
                          frame #2 {
                            n33 = case shown="0, Default" w267 {
                              tunnel: w268 -> [_ w270]
                              frame 0, Default {
                              }
                              frame 1 {
                                n34 = call "I3252_Edit_Setpoint.vi"("Read String"=w270) -> ("Setpoint is"=→"SP 1 is (°C)":dbl)
                              }
                            }
                          }
                        }
                      }
                    }
                    frame #2 {
                      n35 = property on="Setpoint\n START" class="Bool"("Blinking"=FALSE) -> ()  [unwired: 2 in, 2 out]
                    }
                  }
                  n36 = Not(x="Setpoint\n START") -> (.not. x?=w228:bool)
                }
                event "Standby": Value Change {
                  n37 = event-data() -> ()  [unwired: 1 in, 1 out]
                  n38 = flat-sequence {
                    tunnel: [w285] -> w275
                    tunnel: w275 -> [w289]
                    tunnel: w274 -> [w288]
                    tunnel: [w287] -> w272
                    tunnel: [w286] -> w273
                    frame #0 {
                      n39 = local read "Standby"() -> (w278:bool)
                      n40 = Select(t=TRUE, s=w278, f=FALSE) -> (s? t:f=w281:bool)
                      n41 = property on="Standby" class="Bool (strict)"("Blinking"=w281) -> ()  [unwired: 2 in, 2 out]
                    }
                    frame #1 {
                      n42 = local read "Standby"() -> (w283:bool)
                      n43 = Select(t="*D03", s=w283, f="*E03") -> (s? t:f=w285:string)
                    }
                    frame #2 {
                      n44 = Unbundle(w288) -> ("VISA resource name out"=w290:refnum<visa-resource-name>, "error out"=w292:errorcluster, "Delay (ms)"=w291:u32, "Write/\nRead"=w293:bool)
                      n45 = call "I3252_Comm_Interface.vi"("VISA resource name in"=w290, "error in"=w292, "Delay (ms)"=w291, "Write"=w293, "String to Write"=w289, "Read"=w293) -> ("VISA resource name out"=w286:refnum<visa-resource-name>, "error out"=w287:errorcluster)  [unwired: 2 in, 1 out]
                    }
                  }
                  n46 = Not(x="Standby") -> (.not. x?=w277:bool)
                }
                event "Set Command": Value Change {
                  n47 = event-data() -> ()  [unwired: 1 in, 1 out]
                  n48 = stacked-sequence {
                    tunnel: w296 -> [_ w303 _]
                    tunnel: [_ w302 _] -> w295
                    tunnel: [_ w301 _] -> w294
                    frame #0 {
                      n49 = property on="Set Command" class="Bool"("Blinking"=TRUE) -> ()  [unwired: 2 in, 2 out]
                      n50 = property on="Read Temperature" class="Bool (strict)"("Blinking"=FALSE) -> ()  [unwired: 2 in, 2 out]
                    }
                    frame #1 {
                      n51 = flat-sequence {
                        tunnel: [w308] -> w305
                        tunnel: [w311] -> w304
                        tunnel: w305 -> [w312]
                        tunnel: w303 -> [w313]
                        tunnel: [w310] -> w302
                        tunnel: [w309] -> _
                        tunnel: [w309] -> w301
                        tunnel: w304 -> [w318]
                        frame #0 {
                          n52 = Concatenate Strings("*", "Command shall be") -> (w308:string)
                        }
                        frame #1 {
                          n53 = Unbundle(w313) -> ("VISA resource name out"=w317:refnum<visa-resource-name>, "error out"=w315:errorcluster, "Delay (ms)"=w316:u32, "Write/\nRead"=w314:bool)
                          n54 = call "I3252_Comm_Interface.vi"("VISA resource name in"=w317, "error in"=w315, "Delay (ms)"=w316, "Write"=w314, "String to Write"=w312, "Read"=w314) -> ("VISA resource name out"=w310:refnum<visa-resource-name>, "error out"=w309:errorcluster, "Read String"=w311:string)  [unwired: 2 in]
                        }
                        frame #2 {
                          "Command is" <- w318
                        }
                      }
                    }
                    frame #2 {
                      n55 = property on="Set Command" class="Bool"("Blinking"=FALSE) -> ()  [unwired: 2 in, 2 out]
                    }
                  }
                  n56 = Not(x="Set Command") -> (.not. x?=w298:bool)
                }
                event "Reset\nSTOPP": Value Change {
                  n57 = event-data() -> ()  [unwired: 1 in, 1 out]
                  n58 = stacked-sequence {
                    tunnel: [_ w331 _] -> w321
                    tunnel: [_ w330 _] -> w322
                    tunnel: w320 -> [_ w328 _]
                    frame #0 {
                      n59 = property on="Reset\nSTOPP" class="Bool"("Blinking"=TRUE) -> ()  [unwired: 2 in, 2 out]
                      n60 = property on="Read Temperature" class="Bool (strict)"("Blinking"=FALSE) -> ()  [unwired: 2 in, 2 out]
                    }
                    frame #1 {
                      n61 = for {
                        N: 2 -> [_]
                        tunnel: [w337] -> w331
                        tunnel: [w336] -> w330
                        tunnel: w328 -> [w335]
                        i -> [w333]
                        n62 = flat-sequence {
                          tunnel: w333 -> [w339]
                          tunnel: [w338] -> w334
                          tunnel: [w344] -> w337
                          tunnel: [w345] -> w336
                          tunnel: w335 -> [w346]
                          tunnel: w334 -> [w343]
                          tunnel: [w342] -> w332
                          tunnel: w333 -> [w352]
                          tunnel: w332 -> [w351]
                          frame #0 {
                            n63 = case shown="0, Default" w339 {
                              tunnel: ["*Z02" "*G01"] -> w338
                              frame 0, Default {
                              }
                              frame 1 {
                              }
                            }
                          }
                          frame #1 {
                            n64 = Unbundle(w346) -> ("VISA resource name out"=w347:refnum<visa-resource-name>, "error out"=w349:errorcluster, "Delay (ms)"=w348:u32, "Write/\nRead"=w350:bool)
                            n65 = call "I3252_Comm_Interface.vi"("VISA resource name in"=w347, "error in"=w349, "Delay (ms)"=w348, "Write"=w350, "String to Write"=w343, "Read"=w350) -> ("VISA resource name out"=w345:refnum<visa-resource-name>, "error out"=w344:errorcluster, "Read String"=w342:string)  [unwired: 2 in]
                          }
                          frame #2 {
                            n66 = case shown="0, Default" w352 {
                              tunnel: w351 -> [_ w354]
                              frame 0, Default {
                              }
                              frame 1 {
                                n67 = call "I3252_Edit_Setpoint.vi"("Read String"=w354) -> ("Setpoint is"=w353:dbl)
                                n68 = local write "SP 1 is (°C)"(w353) -> ()
                              }
                            }
                          }
                        }
                      }
                      n69 = Wait (ms)(milliseconds to wait=u32 4000) -> ()  [unwired: 1 out]
                    }
                    frame #2 {
                      n70 = property on="Reset\nSTOPP" class="Bool"("Blinking"=FALSE) -> ()  [unwired: 2 in, 2 out]
                    }
                  }
                  n71 = Not(x="Reset\nSTOPP") -> (.not. x?=w324:bool)
                }
                event "Auto Tune": Value Change {
                  n72 = event-data() -> ()  [unwired: 1 in, 1 out]
                  n73 = stacked-sequence {
                    tunnel: w358 -> [_ w365 w410]
                    tunnel: [_ w364 _] -> w357
                    tunnel: [_ w363 _] -> w356
                    frame #0 {
                      n74 = property on="Auto Tune" class="Bool"("Blinking"=TRUE) -> ()  [unwired: 2 in, 2 out]
                      n75 = property on="Read Temperature" class="Bool (strict)"("Blinking"=FALSE) -> ()  [unwired: 2 in, 2 out]
                    }
                    frame #1 {
                      n76 = for {
                        N: 4 -> [_]
                        tunnel: [w370] -> w363
                        tunnel: [w369] -> w364
                        tunnel: w365 -> [w368]
                        i -> [w373]
                        n77 = flat-sequence {
                          tunnel: w373 -> [w375]
                          tunnel: [w374] -> w371
                          tunnel: w371 -> [w390]
                          tunnel: [w389] -> w372
                          tunnel: [w392] -> w370
                          tunnel: [w391] -> w369
                          tunnel: w368 -> [w388]
                          tunnel: w373 -> [w398]
                          tunnel: w372 -> [w397]
                          frame #0 {
                            n78 = case shown="0, Default" w375 {
                              tunnel: ["*V01" w378 "*W0C35" "*Z02"] -> w374
                              frame 0, Default {
                              }
                              frame 1 {
                                n79 = local read "Temperature (°C)"() -> (w377:dbl)
                                n80 = Add(x=20.0, y=w377) -> (x+y=w384:dbl)
                                n81 = Multiply(x=10.0, y=w384) -> (x*y=w381:dbl)
                                n82 = Number To Hexadecimal String(1:i16 5 ("width (-)"), 2:w381) -> (0:w380:string)
                                n83 = Concatenate Strings("*W012", w380) -> (w378:string)
                              }
                              frame 2 {
                                # "35 hex = \n00110101 bin"
                              }
                              frame 3 {
                              }
                            }
                          }
                          frame #1 {
                            n84 = Unbundle(w388) -> ("VISA resource name out"=w396:refnum<visa-resource-name>, "error out"=w394:errorcluster, "Delay (ms)"=w395:u32, "Write/\nRead"=w393:bool)
                            n85 = call "I3252_Comm_Interface.vi"("VISA resource name in"=w396, "error in"=w394, "Delay (ms)"=w395, "Write"=w393, "String to Write"=w390, "Read"=w393) -> ("VISA resource name out"=w392:refnum<visa-resource-name>, "error out"=w391:errorcluster, "Read String"=w389:string)  [unwired: 2 in]
                          }
                          frame #2 {
                            n86 = case shown="0, Default" w398 {
                              tunnel: w397 -> [w400]
                              frame 0, Default {
                                n87 = call <vilib>:"Space Constant.vi"() -> ("String"=w403:string)
                                n88 = Search/Split String(string=w400, search string/char (-)=w403) -> (match + rest of string=w402:string)  [unwired: 1 in, 2 out]
                                n89 = Fract/Exp String To Number(use system decimal point (T)=FALSE, string=w402) -> (number=w399:dbl)  [unwired: 2 in, 1 out]
                                n90 = local write "Temperature (°C)"(w399) -> ()
                              }
                            }
                          }
                        }
                      }
                      n91 = Wait (ms)(milliseconds to wait=u32 45000) -> ()  [unwired: 1 out]
                    }
                    frame #2 {
                      n92 = Unbundle(w410) -> ("VISA resource name out"=w409:refnum<visa-resource-name>, "error out"=w407:errorcluster, "Delay (ms)"=w408:u32, "Write/\nRead"=w406:bool)
                      n93 = property on="Auto Tune" class="Bool"("Blinking"=FALSE) -> ()  [unwired: 2 in, 2 out]
                      n94 = call "I3252_Comm_Interface.vi"("VISA resource name in"=w409, "error in"=w407, "Delay (ms)"=w408, "Write"=w406, "String to Write"="*W01200000", "Read"=w406) -> ()  [unwired: 2 in, 3 out]
                    }
                  }
                  n95 = Not(x="Auto Tune") -> (.not. x?=w359:bool)
                }
                event "Write LOW/HI": Value Change {
                  n96 = event-data() -> ()  [unwired: 1 in, 1 out]
                  n97 = stacked-sequence {
                    tunnel: [_ w420 _] -> w413
                    tunnel: [_ w419 _] -> w412
                    tunnel: w411 -> [_ w418 _]
                    frame #0 {
                      n98 = property on="Write LOW/HI" class="Bool"("Blinking"=TRUE) -> ()  [unwired: 2 in, 2 out]
                      n99 = property on="Read Temperature" class="Bool (strict)"("Blinking"=FALSE) -> ()  [unwired: 2 in, 2 out]
                    }
                    frame #1 {
                      n100 = for {
                        N: 4 -> [_]
                        tunnel: [w424] -> w420
                        tunnel: [w423] -> w419
                        tunnel: w418 -> [w422]
                        i -> [w426]
                        n101 = flat-sequence {
                          tunnel: w426 -> [w428]
                          tunnel: [w429] -> w425
                          tunnel: w425 -> [w443]
                          tunnel: [w444] -> w427
                          tunnel: [w446] -> w424
                          tunnel: [w445] -> w423
                          tunnel: w422 -> [w442]
                          tunnel: w427 -> [w452]
                          tunnel: w426 -> [w451]
                          frame #0 {
                            n102 = case shown="1" w428 {
                              tunnel: [w431 w437 "*R27" "*R28"] -> w429
                              frame 0, Default {
                                n103 = Number To Hexadecimal String(1:i16 2 ("width (-)"), 2:"% LOW shall be") -> (0:w432:string)
                                n104 = Concatenate Strings("*W27", w432) -> (w431:string)
                              }
                              frame 1 {
                                n105 = Number To Hexadecimal String(1:i16 2 ("width (-)"), 2:"% High shall be") -> (0:w438:string)
                                n106 = Concatenate Strings("*W28", w438) -> (w437:string)
                              }
                              frame 2 {
                              }
                              frame 3 {
                              }
                            }
                          }
                          frame #1 {
                            n107 = Unbundle(w442) -> ("VISA resource name out"=w450:refnum<visa-resource-name>, "error out"=w448:errorcluster, "Delay (ms)"=w449:u32, "Write/\nRead"=w447:bool)
                            n108 = call "I3252_Comm_Interface.vi"("VISA resource name in"=w450, "error in"=w448, "Delay (ms)"=w449, "Write"=w447, "String to Write"=w443, "Read"=w447) -> ("VISA resource name out"=w446:refnum<visa-resource-name>, "error out"=w445:errorcluster, "Read String"=w444:string)  [unwired: 2 in]
                          }
                          frame #2 {
                            n109 = case shown="0, Default" w451 {
                              tunnel: w452 -> [_ w456 w460]
                              frame 0, Default {
                              }
                              frame 2 {
                                n110 = String Subset(string=w456, offset (0)=3) -> (substring=w454:string)  [unwired: 1 in]
                                n111 = Hexadecimal String To Number(string=w454) -> (number=→"% LOW is":u32)  [unwired: 2 in, 1 out]
                              }
                              frame 3 {
                                n112 = String Subset(string=w460, offset (0)=3) -> (substring=w458:string)  [unwired: 1 in]
                                n113 = Hexadecimal String To Number(string=w458) -> (number=→"% HIGH is":u32)  [unwired: 2 in, 1 out]
                              }
                            }
                          }
                        }
                      }
                    }
                    frame #2 {
                      n114 = property on="Write LOW/HI" class="Bool"("Blinking"=FALSE) -> ()  [unwired: 2 in, 2 out]
                    }
                  }
                  n115 = Not(x="Write LOW/HI") -> (.not. x?=w415:bool)
                }
                event "Set PID": Value Change {
                  n116 = event-data() -> ()  [unwired: 1 in, 1 out]
                  n117 = stacked-sequence {
                    tunnel: w464 -> [_ w471 _]
                    tunnel: [_ w470 _] -> w463
                    tunnel: [_ w469 _] -> w462
                    frame #0 {
                      n118 = property on="Set PID" class="Bool"("Blinking"=TRUE) -> ()  [unwired: 2 in, 2 out]
                      n119 = property on="Read Temperature" class="Bool (strict)"("Blinking"=FALSE) -> ()  [unwired: 2 in, 2 out]
                    }
                    frame #1 {
                      n120 = for {
                        N: 6 -> [_]
                        tunnel: w471 -> [w475]
                        tunnel: [w474] -> w470
                        tunnel: [w473] -> w469
                        i -> [w477]
                        n121 = flat-sequence {
                          tunnel: w477 -> [w479]
                          tunnel: [w480] -> w476
                          tunnel: w476 -> [w521]
                          tunnel: [w517] -> w478
                          tunnel: w475 -> [w520]
                          tunnel: [w519] -> w473
                          tunnel: [w518] -> w474
                          tunnel: w478 -> [w527]
                          tunnel: w477 -> [w526]
                          frame #0 {
                            n122 = case shown="0, Default" w479 {
                              tunnel: [w487 w495 w503 w505 w509 w513] -> w480
                              frame 0, Default {
                                n123 = local read "RAM"() -> (w481:bool)
                                n124 = Number To Hexadecimal String(1:i16 4 ("width (-)"), 2:"P (PB1) shall be") -> (0:w488:string)
                                n125 = Select(t="*P17", s=w481, f="*W17") -> (s? t:f=w482:string)
                                n126 = Concatenate Strings(w482, w488) -> (w487:string)
                              }
                              frame 1 {
                                n127 = local read "RAM"() -> (w489:bool)
                                n128 = Number To Hexadecimal String(1:i16 4 ("width (-)"), 2:"I ( Reset1) shall be") -> (0:w496:string)
                                n129 = Select(t="*P18", s=w489, f="*W18") -> (s? t:f=w491:string)
                                n130 = Concatenate Strings(w491, w496) -> (w495:string)
                              }
                              frame 2 {
                                n131 = local read "RAM"() -> (w498:bool)
                                n132 = Number To Hexadecimal String(1:i16 4 ("width (-)"), 2:"D (Rate) shall be") -> (0:w504:string)
                                n133 = Select(t="*P19", s=w498, f="*W19") -> (s? t:f=w499:string)
                                n134 = Concatenate Strings(w499, w504) -> (w503:string)
                              }
                              frame 3 {
                                n135 = local read "RAM"() -> (w508:bool)
                                n136 = Select(t="*G17", s=w508, f="*R17") -> (s? t:f=w505:string)
                              }
                              frame 4 {
                                n137 = local read "RAM"() -> (w512:bool)
                                n138 = Select(t="*G18", s=w512, f="*R18") -> (s? t:f=w509:string)
                              }
                              frame 5 {
                                n139 = local read "RAM"() -> (w516:bool)
                                n140 = Select(t="*G19", s=w516, f="*R19") -> (s? t:f=w513:string)
                              }
                            }
                          }
                          frame #1 {
                            n141 = Unbundle(w520) -> ("VISA resource name out"=w525:refnum<visa-resource-name>, "error out"=w523:errorcluster, "Delay (ms)"=w524:u32, "Write/\nRead"=w522:bool)
                            n142 = call "I3252_Comm_Interface.vi"("VISA resource name in"=w525, "error in"=w523, "Delay (ms)"=w524, "Write"=w522, "String to Write"=w521, "Read"=w522) -> ("VISA resource name out"=w518:refnum<visa-resource-name>, "error out"=w519:errorcluster, "Read String"=w517:string)  [unwired: 2 in]
                          }
                          frame #2 {
                            n143 = case shown="0, Default" w526 {
                              tunnel: w527 -> [_ w531 w535 w539]
                              frame 0, Default {
                              }
                              frame 3 {
                                n144 = String Subset(string=w531, offset (0)=3) -> (substring=w529:string)  [unwired: 1 in]
                                n145 = Hexadecimal String To Number(string=w529) -> (number=→"P (PB1) is":u32)  [unwired: 2 in, 1 out]
                              }
                              frame 4 {
                                n146 = String Subset(string=w535, offset (0)=3) -> (substring=w533:string)  [unwired: 1 in]
                                n147 = Hexadecimal String To Number(string=w533) -> (number=→"I ( Reset1) is":u32)  [unwired: 2 in, 1 out]
                              }
                              frame 5 {
                                n148 = String Subset(string=w539, offset (0)=3) -> (substring=w537:string)  [unwired: 1 in]
                                n149 = Hexadecimal String To Number(string=w537) -> (number=→"D (Rate) is":u32)  [unwired: 2 in, 1 out]
                              }
                            }
                          }
                        }
                      }
                    }
                    frame #2 {
                      n150 = property on="Set PID" class="Bool"("Blinking"=FALSE) -> ()  [unwired: 2 in, 2 out]
                    }
                  }
                  n151 = Not(x="Set PID") -> (.not. x?=w466:bool)
                }
                event "Get Values": Value Change {
                  n152 = event-data() -> ()  [unwired: 1 in, 1 out]
                  n153 = stacked-sequence {
                    tunnel: w543 -> [_ w550 _]
                    tunnel: [_ w549 _] -> w542
                    tunnel: [_ w548 _] -> w541
                    frame #0 {
                      n154 = property on="Get Values" class="Bool"("Blinking"=TRUE) -> ()  [unwired: 2 in, 2 out]
                      n155 = property on="Read Temperature" class="Bool (strict)"("Blinking"=FALSE) -> ()  [unwired: 2 in, 2 out]
                    }
                    frame #1 {
                      n156 = for {
                        N: 6 -> [_]
                        tunnel: w550 -> [w554]
                        tunnel: [w553] -> w549
                        tunnel: [w552] -> w548
                        i -> [w556]
                        n157 = flat-sequence {
                          tunnel: w556 -> [w558]
                          tunnel: [w559] -> w555
                          tunnel: w555 -> [w581]
                          tunnel: [w582] -> w557
                          tunnel: w554 -> [w580]
                          tunnel: [w579] -> w552
                          tunnel: [w578] -> w553
                          tunnel: w557 -> [w588]
                          tunnel: w556 -> [w587]
                          frame #0 {
                            n158 = case shown="0, Default" w558 {
                              tunnel: [w562 w566 w570 "*R27" "*R28" w576] -> w559
                              frame 0, Default {
                                n159 = local read "RAM"() -> (w563:bool)
                                n160 = Select(t="*G17", s=w563, f="*R17") -> (s? t:f=w562:string)
                              }
                              frame 1 {
                                n161 = local read "RAM"() -> (w567:bool)
                                n162 = Select(t="*G18", s=w567, f="*R18") -> (s? t:f=w566:string)
                              }
                              frame 2 {
                                n163 = local read "RAM"() -> (w571:bool)
                                n164 = Select(t="*G19", s=w571, f="*R19") -> (s? t:f=w570:string)
                              }
                              frame 3 {
                              }
                              frame 4 {
                              }
                              frame 5 {
                                n165 = local read "RAM"() -> (w577:bool)
                                n166 = Select(t="*G01", s=w577, f="*R01") -> (s? t:f=w576:string)
                              }
                            }
                          }
                          frame #1 {
                            n167 = Unbundle(w580) -> ("VISA resource name out"=w586:refnum<visa-resource-name>, "error out"=w584:errorcluster, "Delay (ms)"=w585:u32, "Write/\nRead"=w583:bool)
                            n168 = call "I3252_Comm_Interface.vi"("VISA resource name in"=w586, "error in"=w584, "Delay (ms)"=w585, "Write"=w583, "String to Write"=w581, "Read"=w583) -> ("VISA resource name out"=w578:refnum<visa-resource-name>, "error out"=w579:errorcluster, "Read String"=w582:string)  [unwired: 2 in]
                          }
                          frame #2 {
                            n169 = case shown="0, Default" w587 {
                              tunnel: w588 -> [w590 w594 w598 w602 w606 w610]
                              frame 0, Default {
                                n170 = String Subset(string=w590, offset (0)=3) -> (substring=w591:string)  [unwired: 1 in]
                                n171 = Hexadecimal String To Number(string=w591) -> (number=w589:u32)  [unwired: 2 in, 1 out]
                                n172 = local write "P (PB1) shall be"(w589) -> ()
                                n173 = local write "P (PB1) is"(w589) -> ()
                              }
                              frame 1 {
                                n174 = String Subset(string=w594, offset (0)=3) -> (substring=w595:string)  [unwired: 1 in]
                                n175 = Hexadecimal String To Number(string=w595) -> (number=w593:u32)  [unwired: 2 in, 1 out]
                                n176 = local write "I ( Reset1) shall be"(w593) -> ()
                                n177 = local write "I ( Reset1) is"(w593) -> ()
                              }
                              frame 2 {
                                n178 = String Subset(string=w598, offset (0)=3) -> (substring=w599:string)  [unwired: 1 in]
                                n179 = Hexadecimal String To Number(string=w599) -> (number=w597:u32)  [unwired: 2 in, 1 out]
                                n180 = local write "D (Rate) shall be"(w597) -> ()
                                n181 = local write "D (Rate) is"(w597) -> ()
                              }
                              frame 3 {
                                n182 = String Subset(string=w602, offset (0)=3) -> (substring=w603:string)  [unwired: 1 in]
                                n183 = Hexadecimal String To Number(string=w603) -> (number=w601:u32)  [unwired: 2 in, 1 out]
                                n184 = local write "% LOW shall be"(w601) -> ()
                                n185 = local write "% LOW is"(w601) -> ()
                              }
                              frame 4 {
                                n186 = String Subset(string=w606, offset (0)=3) -> (substring=w607:string)  [unwired: 1 in]
                                n187 = Hexadecimal String To Number(string=w607) -> (number=w605:u32)  [unwired: 2 in, 1 out]
                                n188 = local write "% High shall be"(w605) -> ()
                                n189 = local write "% HIGH is"(w605) -> ()
                              }
                              frame 5 {
                                n190 = call "I3252_Edit_Setpoint.vi"("Read String"=w610) -> ("Setpoint is"=w609:dbl)
                                n191 = local write "SP 1 is (°C)"(w609) -> ()
                              }
                            }
                          }
                        }
                      }
                    }
                    frame #2 {
                      n192 = property on="Get Values" class="Bool"("Blinking"=FALSE) -> ()  [unwired: 2 in, 2 out]
                    }
                  }
                  n193 = Not(x="Get Values") -> (.not. x?=w545:bool)
                }
                event "RAM": Value Change {
                  n194 = event-data() -> ()  [unwired: 1 in, 1 out]
                  n195 = stacked-sequence {
                    tunnel: w614 -> [_ w621 _]
                    tunnel: [_ w620 _] -> w613
                    tunnel: [_ w619 _] -> w612
                    frame #0 {
                      n196 = property on="RAM" class="Bool (strict)"("Blinking"=TRUE) -> ()  [unwired: 2 in, 2 out]
                      n197 = property on="Read Temperature" class="Bool (strict)"("Blinking"=FALSE) -> ()  [unwired: 2 in, 2 out]
                    }
                    frame #1 {
                      n198 = for {
                        N: 6 -> [_]
                        tunnel: w621 -> [w625]
                        tunnel: [w624] -> w620
                        tunnel: [w623] -> w619
                        i -> [w627]
                        n199 = flat-sequence {
                          tunnel: w627 -> [w629]
                          tunnel: [w630] -> w626
                          tunnel: w626 -> [w649]
                          tunnel: [w650] -> w628
                          tunnel: w625 -> [w653]
                          tunnel: [w652] -> w623
                          tunnel: [w651] -> w624
                          tunnel: w628 -> [w659]
                          tunnel: w627 -> [w658]
                          frame #0 {
                            n200 = case shown="0, Default" w629 {
                              tunnel: [w633 w637 w641 "*R27" "*R28" w647] -> w630
                              frame 0, Default {
                                n201 = local read "RAM"() -> (w634:bool)
                                n202 = Select(t="*G17", s=w634, f="*R17") -> (s? t:f=w633:string)
                              }
                              frame 1 {
                                n203 = local read "RAM"() -> (w638:bool)
                                n204 = Select(t="*G18", s=w638, f="*R18") -> (s? t:f=w637:string)
                              }
                              frame 2 {
                                n205 = local read "RAM"() -> (w642:bool)
                                n206 = Select(t="*G19", s=w642, f="*R19") -> (s? t:f=w641:string)
                              }
                              frame 3 {
                              }
                              frame 4 {
                              }
                              frame 5 {
                                n207 = local read "RAM"() -> (w648:bool)
                                n208 = Select(t="*G01", s=w648, f="*R01") -> (s? t:f=w647:string)
                              }
                            }
                          }
                          frame #1 {
                            n209 = Unbundle(w653) -> ("VISA resource name out"=w657:refnum<visa-resource-name>, "error out"=w655:errorcluster, "Delay (ms)"=w656:u32, "Write/\nRead"=w654:bool)
                            n210 = call "I3252_Comm_Interface.vi"("VISA resource name in"=w657, "error in"=w655, "Delay (ms)"=w656, "Write"=w654, "String to Write"=w649, "Read"=w654) -> ("VISA resource name out"=w651:refnum<visa-resource-name>, "error out"=w652:errorcluster, "Read String"=w650:string)  [unwired: 2 in]
                          }
                          frame #2 {
                            n211 = case shown="0, Default" w658 {
                              tunnel: w659 -> [w661 w665 w669 w673 w677 w681]
                              frame 0, Default {
                                n212 = String Subset(string=w661, offset (0)=3) -> (substring=w662:string)  [unwired: 1 in]
                                n213 = Hexadecimal String To Number(string=w662) -> (number=w660:u32)  [unwired: 2 in, 1 out]
                                n214 = local write "P (PB1) shall be"(w660) -> ()
                                n215 = local write "P (PB1) is"(w660) -> ()
                              }
                              frame 1 {
                                n216 = String Subset(string=w665, offset (0)=3) -> (substring=w666:string)  [unwired: 1 in]
                                n217 = Hexadecimal String To Number(string=w666) -> (number=w664:u32)  [unwired: 2 in, 1 out]
                                n218 = local write "I ( Reset1) shall be"(w664) -> ()
                                n219 = local write "I ( Reset1) is"(w664) -> ()
                              }
                              frame 2 {
                                n220 = String Subset(string=w669, offset (0)=3) -> (substring=w670:string)  [unwired: 1 in]
                                n221 = Hexadecimal String To Number(string=w670) -> (number=w668:u32)  [unwired: 2 in, 1 out]
                                n222 = local write "D (Rate) shall be"(w668) -> ()
                                n223 = local write "D (Rate) is"(w668) -> ()
                              }
                              frame 3 {
                                n224 = String Subset(string=w673, offset (0)=3) -> (substring=w674:string)  [unwired: 1 in]
                                n225 = Hexadecimal String To Number(string=w674) -> (number=w672:u32)  [unwired: 2 in, 1 out]
                                n226 = local write "% LOW shall be"(w672) -> ()
                                n227 = local write "% LOW is"(w672) -> ()
                              }
                              frame 4 {
                                n228 = String Subset(string=w677, offset (0)=3) -> (substring=w678:string)  [unwired: 1 in]
                                n229 = Hexadecimal String To Number(string=w678) -> (number=w676:u32)  [unwired: 2 in, 1 out]
                                n230 = local write "% High shall be"(w676) -> ()
                                n231 = local write "% HIGH is"(w676) -> ()
                              }
                              frame 5 {
                                n232 = call "I3252_Edit_Setpoint.vi"("Read String"=w681) -> ("Setpoint is"=w680:dbl)
                                n233 = local write "SP 1 is (°C)"(w680) -> ()
                              }
                            }
                          }
                        }
                      }
                    }
                    frame #2 {
                      n234 = property on="RAM" class="Bool (strict)"("Blinking"=FALSE) -> ()  [unwired: 2 in, 2 out]
                    }
                  }
                  n235 = Not(x="RAM") -> (.not. x?=w616:bool)
                }
                event "Set Gauge to Zero": Value Change {
                  n236 = event-data() -> ()  [unwired: 1 in, 1 out]
                  n237 = flat-sequence {
                    tunnel: w687 -> [w696]
                    tunnel: w694 -> [w697]
                    tunnel: w687 -> [w698]
                    tunnel: [w698] -> w685
                    tunnel: [w697] -> w684
                    tunnel: [w696] -> w683
                    tunnel: [w700] -> w690
                    tunnel: [w699] -> w689
                    tunnel: [w701] -> w688
                    tunnel: w685 -> [w703]
                    tunnel: w684 -> [w702]
                    tunnel: w683 -> [w701]
                    tunnel: w690 -> [w708]
                    tunnel: w689 -> [w707]
                    tunnel: w688 -> [w706]
                    frame #0 {
                      n238 = property on="Set Gauge to Zero" class="Bool"("Blinking"=TRUE) -> ()  [unwired: 2 in, 2 out]
                    }
                    frame #1 {
                      n239 = call "Pfeiffer_Get_Pressure_Status.vi"("Port"=w703, "Sensor Nr.:"=w702) -> ("Pressure"=w700:dbl)  [unwired: 1 in, 8 out]
                      "Pressure 2 (mbar)" <- w700
                      n240 = call "Pfeiffer_Offset_Display.vi"("Port"=w703, "W/R"=FALSE) -> ("Sensor 1 Get"=w699:dbl)  [unwired: 3 in, 6 out]
                      "Old Offset (mbar)" <- w699
                    }
                    frame #2 {
                      n241 = Add(x=w708, y=w707) -> (x+y=w710:dbl)
                      n242 = call "Pfeiffer_Offset_Display.vi"("Port"=w706, "W/R"=TRUE, "Sensor 1 Set"=w710) -> ("Sensor 1 Get"=→"Current Offset (mbar)":dbl)  [unwired: 2 in, 6 out]
                    }
                    frame #3 {
                      n243 = property on="Set Gauge to Zero" class="Bool"("Blinking"=TRUE) -> ()  [unwired: 2 in, 2 out]
                    }
                  }
                  n244 = Unbundle(w693) -> ("VISA resource name out"=w692:refnum<visa-resource-name>, "error out"=w691:errorcluster)  [unwired: 2 out]
                }
                event "Write to File": Value Change {
                  n245 = event-data() -> ("NewVal"=w716:bool)  [unwired: 1 in]
                  n246 = Unbundle(w719) -> ("VISA resource name out"=w718:refnum<visa-resource-name>, "error out"=w717:errorcluster)  [unwired: 2 out]
                  n247 = local read "File Path"() -> (w712:path)
                  n248 = case shown="True" w716 {
                    tunnel: w712 -> [_ w724]
                    tunnel: "User" -> [_ w723]
                    tunnel: "Sample" -> [_ w722]
                    tunnel: [path "" ("File Path") w721] -> w713
                    frame False {
                    }
                    frame True {
                      n249 = call "Header.vi"("Sample"=w722, "User"=w723, "File Path"=w724) -> ("File Path"=w721:path)
                    }
                  }
                  n250 = local write "File Path"(w713) -> ()
                }
              }
            }
            n251 = Bundle(cluster=w211, "VISA resource name out"=w210, "error out"=w209) -> (w208:T9)  [unwired: 2 in]
          }
          frame #1 {
            n252 = Unbundle(w735) -> ("Delay (ms)"=w734:u32)  [unwired: 3 out]
            n253 = Multiply(x="Intervall (s)", y=u32 1000) -> (x*y=w732:u32)
            n254 = Subtract(x=w732, y=w734) -> (x-y=w731:u32)
            n255 = Wait (ms)(milliseconds to wait=w731) -> ()  [unwired: 1 out]
          }
          frame #2 {
            (unwired) "Daniel Schuster (geb. 20.03.1988)"
            n256 = node-c288(w773) -> (w779:T5)  [unwired: 2 in]
            n257 = node-c288(w760) -> (w762:T5)  [unwired: 2 in]
            n258 = node-c288(w755) -> (w765:T5)  [unwired: 2 in]
            n259 = node-c288(w774) -> (w777:T5)  [unwired: 2 in]
            n260 = node-c288(w772) -> (w783:T5)  [unwired: 2 in]
            n261 = timed-sequence {
              timing: w779 -> [_]
              timing-out: [_] -> w778
              tunnel: w775 -> [w863]
              tunnel: [w862] -> w769
              tunnel: [w861] -> w768
              tunnel: [w860] -> w750
              n262 = timed-flat-sequence {
                tunnel: w863 -> [w867]
                tunnel: [w866] -> w862
                tunnel: [w865] -> w861
                tunnel: [w864] -> w860
                n263 = node-c288() -> ()  [unwired: 1 in, 1 out]
                n264 = case shown="True" "Read Temperature" {
                  tunnel: w867 -> [w871 w876]
                  tunnel: [w870 w875] -> w866
                  tunnel: [w869 w874] -> w865
                  tunnel: [_ w873] -> w864
                  frame False {
                    n265 = Unbundle(w871) -> ("VISA resource name out"=w870:refnum<visa-resource-name>, "error out"=w869:errorcluster)  [unwired: 2 out]
                    n266 = property on="Read Temperature" class="Bool (strict)"("Blinking"=FALSE) -> ()  [unwired: 2 in, 2 out]
                  }
                  frame True {
                    n267 = stacked-sequence {
                      tunnel: w876 -> [_ w881]
                      tunnel: [_ w880] -> w875
                      tunnel: [_ w879] -> w874
                      tunnel: [_ w878] -> w873
                      frame #0 {
                        n268 = property on="Read Temperature" class="Bool (strict)"("Blinking"=TRUE) -> ()  [unwired: 2 in, 2 out]
                      }
                      frame #1 {
                        n269 = Unbundle(w881) -> ("VISA resource name out"=w885:refnum<visa-resource-name>, "error out"=w883:errorcluster, "Delay (ms)"=w884:u32, "Write/\nRead"=w882:bool)
                        n270 = call "I3252_Comm_Interface.vi"("VISA resource name in"=w885, "error in"=w883, "Delay (ms)"=w884, "Write"=w882, "String to Write"="*V01", "Read"=w882) -> ("VISA resource name out"=w880:refnum<visa-resource-name>, "error out"=w879:errorcluster, "Read String"=w878:string)  [unwired: 2 in]
                      }
                    }
                  }
                }
                n271 = node-c288() -> ()  [unwired: 1 in, 1 out]
              }
            }
            n272 = timed-sequence {
              timing: w762 -> [_]
              timing-out: [_] -> w761
              tunnel: w759 -> [w788]
              tunnel: w758 -> [w787]
              tunnel: [w786] -> w756
              tunnel: [w785] -> w757
              tunnel: [w784] -> w752
              n273 = timed-flat-sequence {
                tunnel: w788 -> [w793]
                tunnel: w787 -> [w792]
                tunnel: [w791] -> w786
                tunnel: [w790] -> w785
                tunnel: [w789] -> w784
                n274 = node-c288() -> ()  [unwired: 1 in, 1 out]
                n275 = case shown="True" "Read VC 840 2" {
                  tunnel: w793 -> [w797 w803]
                  tunnel: w792 -> [w798 w802]
                  tunnel: [w797 w801] -> w791
                  tunnel: [w798 w800] -> w790
                  tunnel: [0.0 ("Reading") w799] -> w789
                  frame False {
                    n276 = property on="Read VC 840 2" class="Bool (strict)"("Blinking"=FALSE) -> ()  [unwired: 2 in, 2 out]
                  }
                  frame True {
                    n277 = stacked-sequence {
                      tunnel: w803 -> [_ w810]
                      tunnel: w802 -> [_ w809]
                      tunnel: [_ w808] -> w801
                      tunnel: [_ w807] -> w800
                      tunnel: [_ w805] -> w799
                      frame #0 {
                        n278 = property on="Read VC 840 2" class="Bool (strict)"("Blinking"=TRUE) -> ()  [unwired: 2 in, 2 out]
                      }
                      frame #1 {
                        n279 = call "VC840_Read.vi"("error in (no error)"=w809, "VISA resource name"=w810) -> ("error out"=w807:errorcluster, "Unit"=→"Unit 2":string, "Reading"=w805:dbl, "VISA resource name out"=w808:refnum<visa-resource-name>, "Status"=→"Status 2":T4, "Mode"=→"Mode 2":enum16{"?", "Diode", "Beep", "DC", "AC"})  [unwired: 4 out]
                        "Reading 2" <- w805
                      }
                    }
                  }
                }
                n280 = node-c288() -> ()  [unwired: 1 in, 1 out]
              }
            }
            n281 = timed-sequence {
              timing: w765 -> [_]
              timing-out: [_] -> w764
              tunnel: w767 -> [w822]
              tunnel: w766 -> [w821]
              tunnel: [w820] -> w763
              tunnel: [w819] -> w751
              n282 = timed-flat-sequence {
                tunnel: w822 -> [w826]
                tunnel: w821 -> [w825]
                tunnel: [w824] -> w820
                tunnel: [w823] -> w819
                n283 = node-c288() -> ()  [unwired: 1 in, 1 out]
                n284 = case shown="True" "Read Pressure" {
                  tunnel: w826 -> [_ w831]
                  tunnel: w825 -> [_ w832]
                  tunnel: [_ w833] -> w824
                  tunnel: [0.0 ("Pressure") w830] -> w823
                  frame False {
                    n285 = property on="Read Pressure" class="Bool (strict)"("Blinking"=FALSE) -> ()  [unwired: 2 in, 2 out]
                  }
                  frame True {
                    n286 = stacked-sequence {
                      tunnel: [_ w839] -> w833
                      tunnel: w832 -> [_ w838]
                      tunnel: w831 -> [_ w837]
                      tunnel: [_ w835] -> w830
                      frame #0 {
                        n287 = property on="Read Pressure" class="Bool (strict)"("Blinking"=TRUE) -> ()  [unwired: 2 in, 2 out]
                      }
                      frame #1 {
                        n288 = call "Pfeiffer_Get_Pressure_Status.vi"("Port"=w838, "Sensor Nr.:"=w837) -> ("Pressure"=w835:dbl, "Status"=→"Status":i32, "Error Out"=w839:bool)  [unwired: 7 in]
                        "Pressure 1 (mbar)" <- w835
                        "Pressure (mbar)" <- w835
                      }
                    }
                  }
                }
                n289 = node-c288() -> ()  [unwired: 1 in, 1 out]
              }
            }
            n290 = timed-sequence {
              timing: w777 -> [_]
              timing-out: [_] -> w776
              tunnel: [w846] -> w754
              n291 = timed-flat-sequence {
                tunnel: [w847] -> w846
                w848 = 10.0 ("y")
                n292 = node-c288() -> ()  [unwired: 1 in, 1 out]
                n293 = call "System_Time_in_Seconds.vi"() -> ("Current Time (s)"=w853:dbl)
                n294 = local read "Starttime"() -> (w852:dbl)
                n295 = Subtract(x=w853, y=w852) -> (x-y=w850:dbl)
                n296 = Multiply(x=w850, y=w848) -> (x*y=w851:dbl)
                n297 = Round To Nearest(number=w851) -> (nearest integer value=w849:dbl)
                n298 = Divide(x=w849, y=w848) -> (x/y=w847:dbl)
                "time (s)" <- w847
                n299 = node-c288() -> ()  [unwired: 1 in, 1 out]
              }
            }
            n300 = timed-sequence {
              timing: w783 -> [_]
              timing-out: [_] -> w782
              tunnel: w781 -> [w897]
              tunnel: w780 -> [w896]
              tunnel: [w895] -> w771
              tunnel: [w894] -> w770
              tunnel: [w893] -> w753
              n301 = timed-flat-sequence {
                tunnel: w897 -> [w902]
                tunnel: w896 -> [w901]
                tunnel: [w900] -> w895
                tunnel: [w899] -> w894
                tunnel: [w898] -> w893
                n302 = node-c288() -> ()  [unwired: 1 in, 1 out]
                n303 = case shown="True" "Read VC 840 1" {
                  tunnel: w902 -> [w906 w912]
                  tunnel: w901 -> [w907 w911]
                  tunnel: [w906 w910] -> w900
                  tunnel: [w907 w909] -> w899
                  tunnel: [0.0 ("Reading") w908] -> w898
                  frame False {
                    n304 = property on="Read VC 840 1" class="Bool (strict)"("Blinking"=FALSE) -> ()  [unwired: 2 in, 2 out]
                  }
                  frame True {
                    n305 = stacked-sequence {
                      tunnel: w912 -> [_ w919]
                      tunnel: w911 -> [_ w918]
                      tunnel: [_ w917] -> w910
                      tunnel: [_ w916] -> w909
                      tunnel: [_ w914] -> w908
                      frame #0 {
                        n306 = property on="Read VC 840 1" class="Bool (strict)"("Blinking"=TRUE) -> ()  [unwired: 2 in, 2 out]
                      }
                      frame #1 {
                        n307 = call "VC840_Read.vi"("error in (no error)"=w918, "VISA resource name"=w919) -> ("error out"=w916:errorcluster, "Unit"=→"Unit 1":string, "Reading"=w914:dbl, "VISA resource name out"=w917:refnum<visa-resource-name>, "Status"=→"Status 1":T4, "Mode"=→"Mode 1":enum16{"?", "Diode", "Beep", "DC", "AC"})  [unwired: 4 out]
                        "Reading 1" <- w914
                      }
                    }
                  }
                }
                n308 = node-c288() -> ()  [unwired: 1 in, 1 out]
              }
            }
            n309 = node-c288(w764) -> ()  [unwired: 1 out]
            n310 = node-c288(w782) -> ()  [unwired: 1 out]
            n311 = node-c288(w761) -> ()  [unwired: 1 out]
            n312 = node-c288(w778) -> ()  [unwired: 1 out]
            n313 = node-c288(w776) -> ()  [unwired: 1 out]
          }
          frame #3 {
            n314 = Build Array (concatenate)(w947, w946) -> (w945:dbl[])
            n315 = Greater?(x=w946, y="Pressure Limit (mbar)") -> (0:w950:bool)
            n316 = case shown="True" w950 {
              frame False {
                n317 = property on="Standby" class="Bool (strict)"("DisabledEnum"=T8."Enabled" ("Disabled")) -> ()  [unwired: 2 in, 2 out]
              }
              frame True {
                n318 = property on="Standby" class="Bool (strict)"("Val(Sgnl)"=TRUE ("Standby"), "DisabledEnum"=T8."Disabled" ("Disabled")) -> ()  [unwired: 2 in, 2 out]
              }
            }
            n319 = call "Resistivity_Calculation.vi"("Reading 1 (V)"=w938, "Constant"="Constant", "Thickness (nm)"="Thickness (nm)", "Reading 2 (A)"=w948) -> ("Resivtivity (Ohm*cm)"=w930:dbl, "Current"=w931:dbl, "Voltage"=w932:dbl)
            "Resistivity (Ohm*cm)" <- w930
            "Voltage (V)" <- w932
            "Current (A)" <- w931
            n320 = call "I3252_Edit_Temperature.vi"("Temp. String"=w949) -> ("Temp. (°C)"=w941:dbl)
            "Temperature (°C)" <- w941
            n321 = Build Array (concatenate)(w943, w944) -> (w940:dbl[])
            n322 = Build Array (concatenate)(w942, w941) -> (w928:dbl[])
            n323 = Build Array (concatenate)(w939, w932) -> (w937:dbl[])
            n324 = Build Array (concatenate)(w936, w931) -> (w934:dbl[])
            n325 = Build Array (concatenate)(w935, w930) -> (w933:dbl[])
            n326 = Build Array(w932, w931, w930) -> (w929:dbl[])
          }
          frame #4 {
            n327 = Bundle(w967, w976) -> (→"Pressure":cluster{dbl[], dbl[]})  [unwired: 1 in]
            n328 = Bundle(w967, w966) -> (→"Temperature":cluster{dbl[], dbl[]})  [unwired: 1 in]
            n329 = Bundle(w967, w969) -> (→"Voltage":cluster{dbl[], dbl[]})  [unwired: 1 in]
            n330 = Bundle(w967, w970) -> (→"Current":cluster{dbl[], dbl[]})  [unwired: 1 in]
            n331 = Bundle(w967, w971) -> (→"Resistivity":cluster{dbl[], dbl[]})  [unwired: 1 in]
            n332 = Build Array (concatenate)(w965, w978, w977, w964) -> (w986:dbl[])
            "appended array" <- w986
          }
          frame #5 {
            n333 = case shown="True" "Write to File" {
              tunnel: [_ w1011] -> w996
              tunnel: "File Path" -> [_ w1009]
              tunnel: w988 -> [_ w1007]
              frame False {
                n334 = property on="Write to File" class="Bool (strict)"("Blinking"=FALSE) -> ()  [unwired: 2 in, 2 out]
              }
              frame True {
                n335 = flat-sequence {
                  tunnel: [w1013] -> w1010
                  tunnel: w1009 -> [w1013]
                  tunnel: [w1012] -> w1008
                  tunnel: w1007 -> [w1012]
                  tunnel: [w1018] -> w1011
                  tunnel: w1010 -> [w1017]
                  tunnel: w1008 -> [w1016]
                  frame #0 {
                    n336 = property on="Write to File" class="Bool (strict)"("Blinking"=TRUE) -> ()  [unwired: 2 in, 2 out]
                  }
                  frame #1 {
                    n337 = call-poly <vilib>:"Write To Spreadsheet File.vi"("format (%.3f)"="%g", "append to file? (new file:F)"=TRUE ("transpose? (no:F)"), "1D data"=w1016, "file path (dialog if empty)"=w1017) -> ("new file path (Not A Path if cancelled)"=w1018:path)  [unwired: 4 in]
                  }
                }
              }
            }
            n338 = Merge Errors(w1001, w1000, w998) -> (w999:errorcluster)
            n339 = call <vilib>:"Simple Error Handler.vi"("error in (no error)"=w999) -> ("error?"=w987:bool)  [unwired: 4 in, 4 out]
            n340 = local write "File Path"(w996) -> ()
          }
        }
      }
    }
    frame #4 {
      n341 = call "VC840_Close.vi"("error in (no error)"=w1022, "VISA resource name"=w1023) -> ("error out"=w1031:errorcluster)  [unwired: 9 in]
      n342 = call "VC840_Close.vi"("error in (no error)"=w1024, "VISA resource name"=w1025) -> ("error out"=w1029:errorcluster)  [unwired: 9 in]
      n343 = VISA Close(VISA resource name=w1027, error in (no error)=w1026) -> (error out=w1028:errorcluster)
      n344 = Merge Errors(w1028, w1029, w1031) -> (w1030:errorcluster)
      n345 = call <vilib>:"Simple Error Handler.vi"("error in (no error)"=w1030) -> ("error?"=w1020:bool)  [unwired: 1 in, 7 out]
      n346 = Stop(stop? (T)=w1020) -> ()
      "Error Out" <- w1021
    }
  }
